vi "POM_PROM_host(1).vi"() -> ()   [LabVIEW 2013]
uses:
  <instrlib>/niDMM/nidmm.llb/niDMM Resolution in Digits.ctl
  <instrlib>/niDMM/nidmm.llb/niDMM Function.ctl
  <instrlib>/niDCPower/nidcpower.llb/niDCPower Measurement Type.ctl
  <vilib>/Analysis/baseanly.llb/Mean (DBL).vi
  <instrlib>/niDMM/nidmm.llb/niDMM Configure Measurement Digits.vi
  <vilib>/Analysis/NI_AALBase.lvlib
panel:
  in  "Принудительная стабилизация":bool
  out "I_pd, uA":dbl=291.5740420576185
  out "IPD(ext), mA":dbl=5.462609109167353
  out "IPD, mA":dbl(graph)=5.462609109167353
  out "Использовать Офир?":bool
  out "Monitor Current, uA":dbl(graph)=291.5700024459511
  in  "В ручную":bool
  in  "Напряжение Пельтье":dbl=0.8
  in  "Нагрев":bool
  in  "№#":i32=1802001
  out "Стабилизировано":bool=TRUE
  in  "+ V TEC для новой точки":dbl=0.11 format="%#_13g"
  in  "Вычет для \"антиразгона\"":dbl format="%#_13g"
  in  "Оставить в раб.\nрежиме":bool
  out "Boolean":bool
  in  "Num_hits_req":u64=5
  out "Num_hits":u64=371
  in  "Count_hits?":bool
  in  "tstab между точками, мс":u32=1
  in  "Предел тока PDext, мА":dbl=20.0
  in  "Dose":i32=7
  in  "Отладка(F)/\n/Рабочий(T)":bool=TRUE
  out "TEC_current, mA":dbl=186.4027731461029
  out "V2(Ild)_Log_address":refnum<file>
  out "Ipd(Ild)_External_Log_address":refnum<file>
  in  "Param_Log":path=path "D:/#rkm/Фонон-4/ТермоЛазер/Фонон-4_ПОМ_ПрОМ/Прога/Updated/ThermoLaser/Logs/Проверка/Проверка"
  out "Param_Log_address":refnum<file>
  out "Op(Ild)_Log_address":refnum<file>
  out "Ipd(Ild)_Monitor_Log_address":refnum<file>
  in  "trelax":u32=35000
  out "Volt_onRes":dbl=2.2062080678161866
  out "NoStab":bool
  out "Operating Current, mA":dbl=47.943356447720134
  in  "Desirable Operating current, mA":dbl=48.0 format="%#_6f"
  out "Error message":string
  in  "Up_Volt_limit":dbl=5.0
  in  "Low_Volt_limit":dbl=1.0
  out "ThRes_stabil":bool=TRUE
  out "Подстроенное напряжение\nстабилизации":dbl=0.7127853808593756
  out "ThRes value":dbl=17929.437890625
  in  "Optimum ThRes":dbl=18000.0 format="%#_6f"
  in  "Предел тока LD, мА":dbl=70.0
  in  "Предел тока ТЕС, мА":dbl=300.0
  in  "Tab Control":enum32{"Page 1", "Page 2", "Page 3", "Page 4"}(tab)=enum."Page 4"
  out "RES(U_TEC) Graph":cluster{dbl[], dbl[]}(graph)={[-0.0, 0.025, 0.05, 0.07500000000000001, 0.1, 0.125, 0.15, 0.175, 0.19999999999999998, 0.22499999999999998, 0.24999999999999997, 0.27499999999999997, 0.3, 0.325, 0.35000000000000003, 0.37500000000000006, 0.4000000000000001, 0.4250000000000001, 0.4500000000000001, 0.47500000000000014, 0.5000000000000001, 0.5250000000000001, 0.5500000000000002, 0.5750000000000002, 0.6000000000000002, 0.6250000000000002, 0.6500000000000002, 0.6750000000000003, 0.7000000000000003, 0.7250000000000003, 0.7500000000000003, 0.7750000000000004], [15319.04365234375, 15328.19267578125, 15358.49169921875, 15409.562109375, 15479.3826171875, 15563.1861328125, 15668.50888671875, 15780.12734375, 15906.40224609375, 16043.244921875, 16186.97255859375, 16341.84609375, 16507.0697265625, 16676.522265625, 16856.963671875, 17044.884375, 17239.0294921875, 17436.3736328125, 17641.744140625, 17850.8728515625, 18071.7896484375, 18291.20625, 18518.965625, 18750.4271484375, 18987.4517578125, 19230.0744140625, 19480.026171875, 19731.8517578125, 19984.940234375, 20249.54140625, 20514.206640625, 20780.055078125]}
  out "RES(I_TEC) Graph":cluster{dbl[], dbl[]}(graph)={[0.03457500435386299, 4.049114950716204, 7.9212407853678135, 11.611043015146826, 15.078954849250364, 18.53827902856892, 21.88408259580828, 25.295266856430793, 28.546483256934756, 31.60504570629327, 34.77027313644012, 37.80993408960394, 40.856486299311584, 43.94949565069024, 47.03219408159836, 50.06845592920464, 52.92926046093485, 55.95350027659507, 58.865931959242474, 61.84202368829837, 64.7802788203752, 67.60156326899994, 70.44177990185035, 73.41963022613506, 76.46974363403558, 79.22741287887104, 82.2001312992484, 85.07135997639818, 88.0785044464861, 90.98931976346292, 93.95691599392462, 96.75420696595256], [15319.04365234375, 15328.19267578125, 15358.49169921875, 15409.562109375, 15479.3826171875, 15563.1861328125, 15668.50888671875, 15780.12734375, 15906.40224609375, 16043.244921875, 16186.97255859375, 16341.84609375, 16507.0697265625, 16676.522265625, 16856.963671875, 17044.884375, 17239.0294921875, 17436.3736328125, 17641.744140625, 17850.8728515625, 18071.7896484375, 18291.20625, 18518.965625, 18750.4271484375, 18987.4517578125, 19230.0744140625, 19480.026171875, 19731.8517578125, 19984.940234375, 20249.54140625, 20514.206640625, 20780.055078125]}
  out "I_PD_Ext(I_LD) Graph":cluster{dbl[], dbl[]}(graph)={[0.0, 5.125820672560687, 10.202363077068034, 15.09070291650038, 20.026524721844005, 24.848748653112324, 29.706585438813228, 34.55255888002156, 39.41379829521783, 44.31743313126964, 49.35841653002704], [0.6213749657825949, 0.6126206411732633, 0.5986137214569519, 0.5846068013204628, 0.5933611264550083, 0.5670981505590477, 0.5355825775341941, 0.586357666360488, 0.5355825775341941, 0.5478386339632713, 0.5390843079753067]}
  out "I_PD(I_LD) Graph":cluster{dbl[], dbl[]}(graph)={[0.0, 5.125820672560687, 10.202363077068034, 15.09070291650038, 20.026524721844005, 24.848748653112324, 29.706585438813228, 34.55255888002156, 39.41379829521783, 44.31743313126964, 49.35841653002704], [0.00446055423708458, 0.1890051237296575, 1.3185992656872259, 47.69851657329127, 96.3842059718445, 145.3466946259141, 195.95923949964345, 243.1108383461833, 288.08951028622687, 334.6654470078647, 377.8655605856329]}
  out "I_pd, uA 2":dbl
  out "V2(I_LD) Graph":cluster{dbl[], dbl[]}(graph)={[0.0, 5.125820672560687, 10.202363077068034, 15.09070291650038, 20.026524721844005, 24.848748653112324, 29.706585438813228, 34.55255888002156, 39.41379829521783, 44.31743313126964, 49.35841653002704], [0.0006418486043783589, 1.1699665507043246, 1.452329111789965, 1.6798119558569469, 1.9201177244634586, 2.150803801269446, 2.3862573437846697, 2.612869753183121, 2.8439823589319366, 3.0683008415602466, 3.3013683877429134]}
  out "Forward Voltage, V":dbl
  out "OP(I_LD) Graph":cluster{dbl[], dbl[]}(graph)={[0.0, 5.125820672560687, 10.202363077068034, 15.09070291650038, 20.026524721844005, 24.848748653112324, 29.706585438813228, 34.55255888002156, 39.41379829521783, 44.31743313126964, 49.35841653002704], [0.0, 0.0, 0.02, 0.74, 1.5, 2.27, 3.0300000000000002, 3.8, 4.58, 5.33, 6.119999999999999]}
  out "Ophir, mW":dbl
  out "Пороговый ток":dbl
  out "Boolean 2":bool
  out "Сопротивление терморез-ра":dbl(graph)=16035.80078125
  out "thRes_adj":dbl=16035.80078125 format="%0.2f"
  in  "Source-Ohm w8":u32=1000
  in  "Coeff_High":dbl=90000.0 format="%#_13g"
  in  "Coeff_low":dbl=20000.0 format="%#_13g"
  in  "Coeff_thr":dbl=1500.0
  out "+Voltage\nrequired":dbl=0.0008410915798611111
  out "Разница ThRes":dbl=75.6982421875
  out "Operating Current":dbl(graph)=0.04003745256828817
  out "Optical Power":dbl(graph)
  out "accommodated voltage (out)":dbl=5.841436967760056
  in  "4070_Rele_source":enum16{"S2_Ch0", "S1_Ch2"}(ring)
  in  "the upper limit for the voltage_LD":dbl=6.0
  in  "the lower limit for the voltage_LD":dbl=1.0
  in  "Start voltage_LD":dbl=2.0 format="%#.7f"
  in  "accuracy_LD":dbl=0.01 step=0.01
  in  "Res_LD":dbl=50.0
  out "#Итерации":i32=31
  in  "TEC_Source":enum16{"S1_Ch2", "S2_Ch0", "S3_Ch1"}(ring)
  in  "Start voltage":dbl=0.1 format="%#.7f"
  in  "the upper limit for the voltage":dbl=1.2
  in  "the lower limit for the voltage":dbl
  in  "Точность ThRes":dbl=75.0 step=0.01
  out "Ro, Ом":dbl=15321.56484375
  in  "OphirLMMeasurementLib.ICoLMMeasurement":refnum<k7>
  out "hDevice":i32=1001
  out "Ophir_address":refnum<k7>
  in  "Power Enable":bool
  in  "4071(2)":refnum<k15>="PXI1Slot4_2"
  out "4071(2)_adress":refnum<k15>="PXI1Slot4_2 (12)" caption="4071(1)_out"
  in  "4071(1)":refnum<k15>="PXI1Slot5_2"
  out "4071(1)_adress":refnum<k15>="PXI1Slot5_2 (12)" caption="4071(1)_out"
  out "4070_address":refnum<k15>="PXI1Slot4_2 (12)" caption="4070_out"
  in  "4070":refnum<k15>="PXI1Slot4_2"
  in  "Source_3":refnum<k15>
  out "Source_3_Vcc_out":refnum<k15> caption="S_3_out"
  out "Source_2_Vcc_out":refnum<k15>="PXI1Slot6 (1)" caption="S_2_out"
  in  "Source_2":refnum<k15>="PXI1Slot6"
  out "Source_1_Vcc_out":refnum<k15>="PXI1Slot2_2 (1)" caption="S_1_out"
  in  "Source_1":refnum<k15>="PXI1Slot2_2"
  out "Прервать":bool=TRUE
  in  "milliseconds to wait":u32=2000
  in  "Шаг напр\nдля TEC, В":dbl=0.025
  in  "Начальное\nнапряжение TEC, В":dbl
  in  "кол-во точек для TEC":i32=32
  in  "stop":bool
  in  "Case":T1(ring)=enum."Quit"
  out "Выполняется":bool
  in  "Раб. режим LD":bool
  in  "Хар-ка TEC":bool
  in  "Хар-ки от I_LD":bool
  out "Status:":string="IDLE"
  out "Подстроенный ток, mA":dbl=43.94711423439531
  in  "Шаг, мА":dbl=5.0
  in  "Начальный ток, мА":dbl
  in  "Кол-во точек":i32=10
  # "20"
  # "7"
  # "5"
  # "0,15"
  # "Охлаждение"
  # "ток Пельтье во время стабилизации"
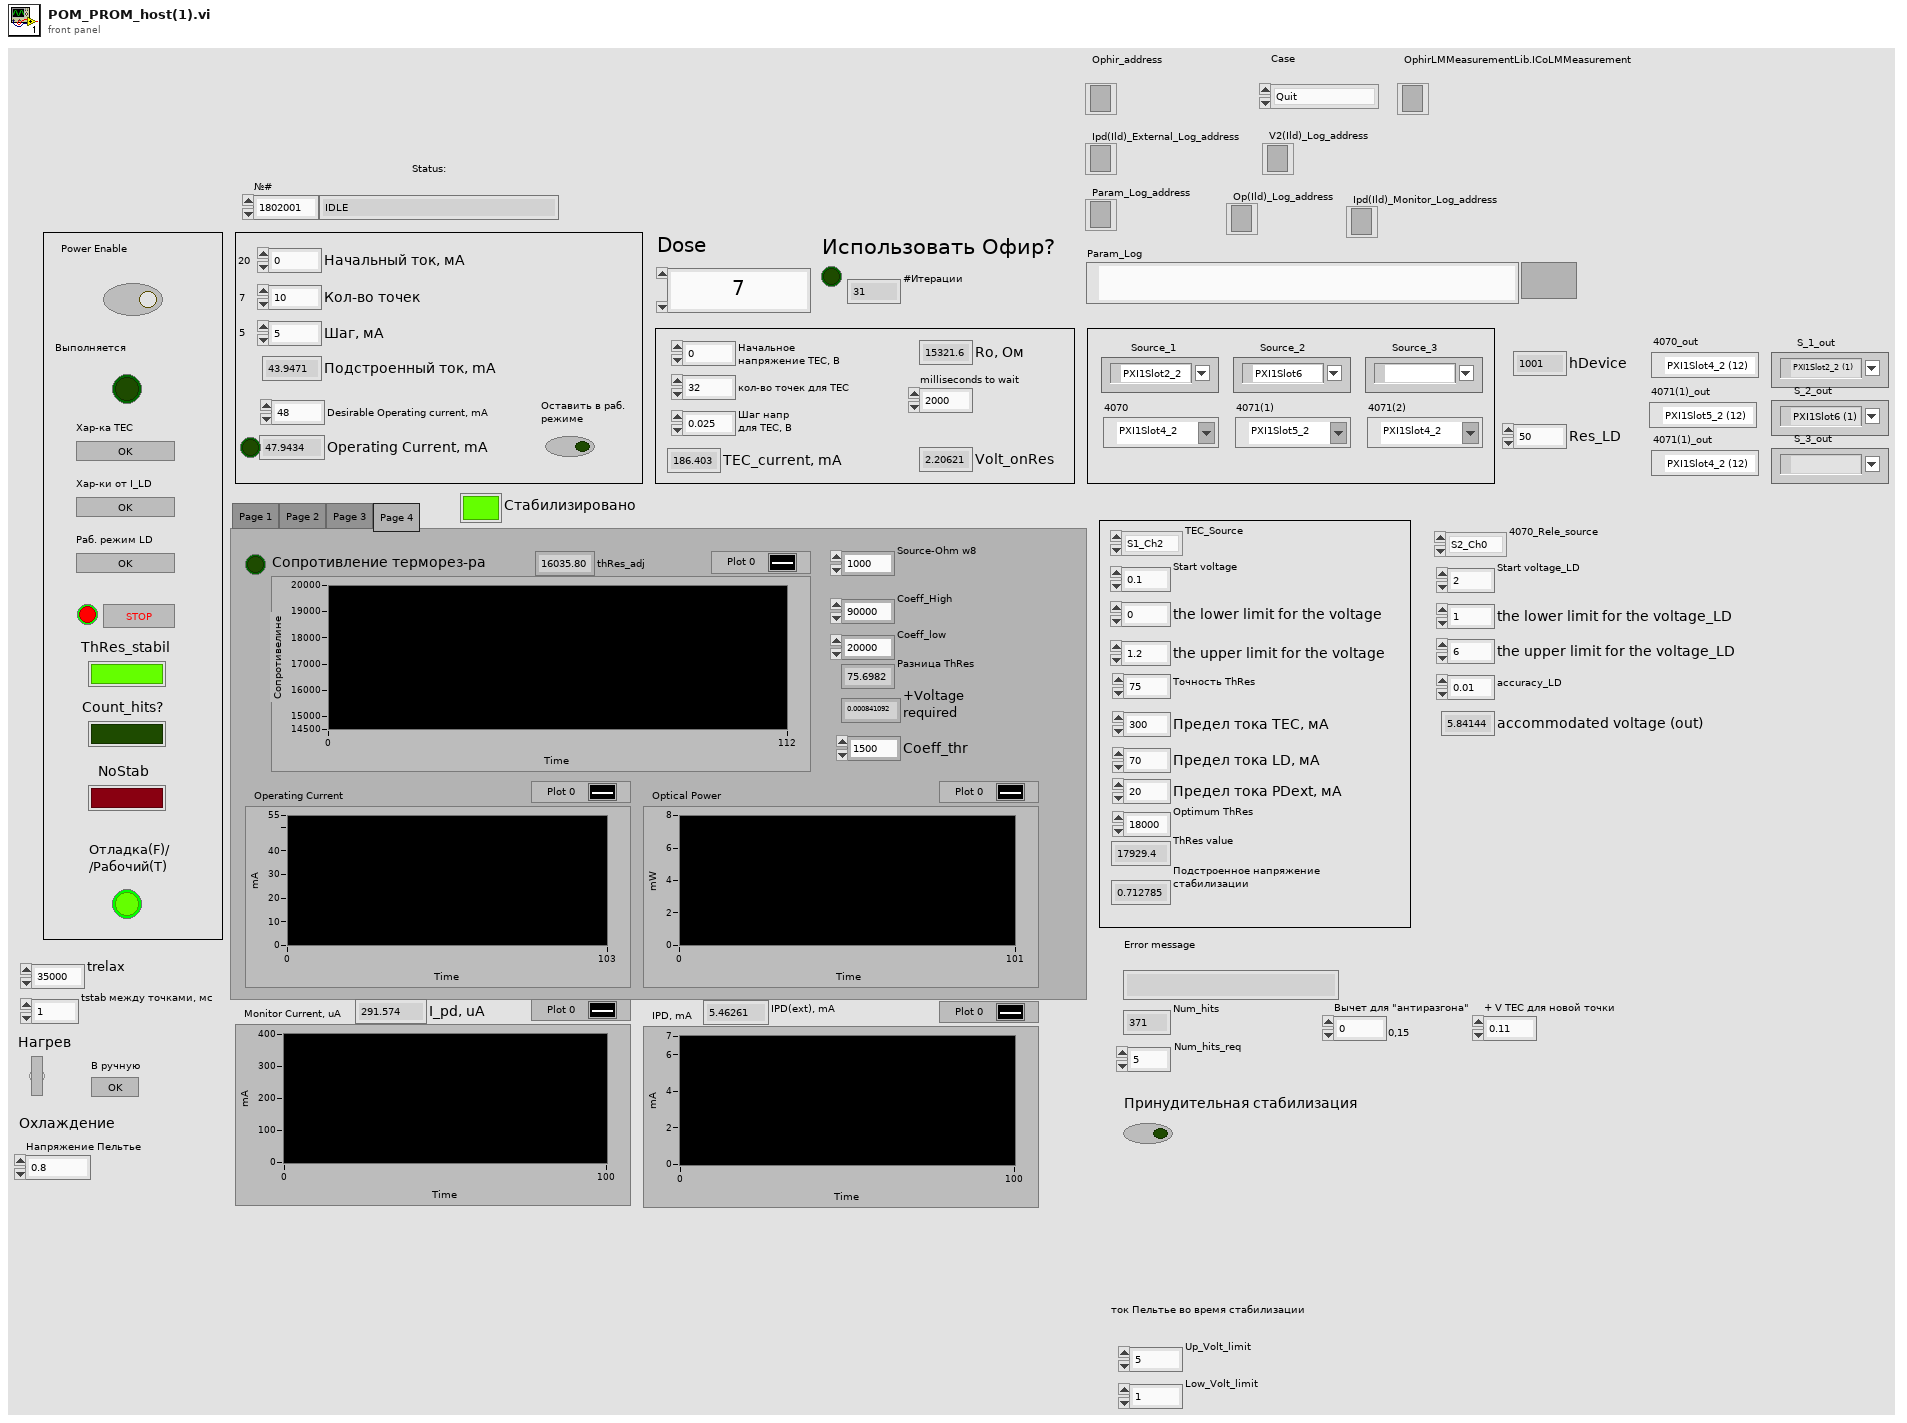
[diagram p1: front panel]
types:
  T1 = enum16{"Initialization", "TEC_Chars", "TRes_Check(Idle)", "Characteristics", "Bias", "Quit"}
  T2 = typedef "niDMM Function.ctl" = enum16{"DC Volts", "AC Volts", "DC Current", "AC Current", "2-wire Resistance", "4-wire Resistance", "Diode", "Frequency", "Period", "AC Volts DC Coupled", "Capacitance", "Inductance", "Temperature"}
  T3 = enum8{"Enabled", "Disabled", "Disabled and Grayed Out"}
  T4 = typedef "niDMM Resolution in Digits.ctl" = dbl
  T5 = enum16{"open", "replace", "create", "open or create", "replace or create", "replace or create with confirmation"}
  T6 = typedef "niDCPower Measurement Type.ctl" = i32
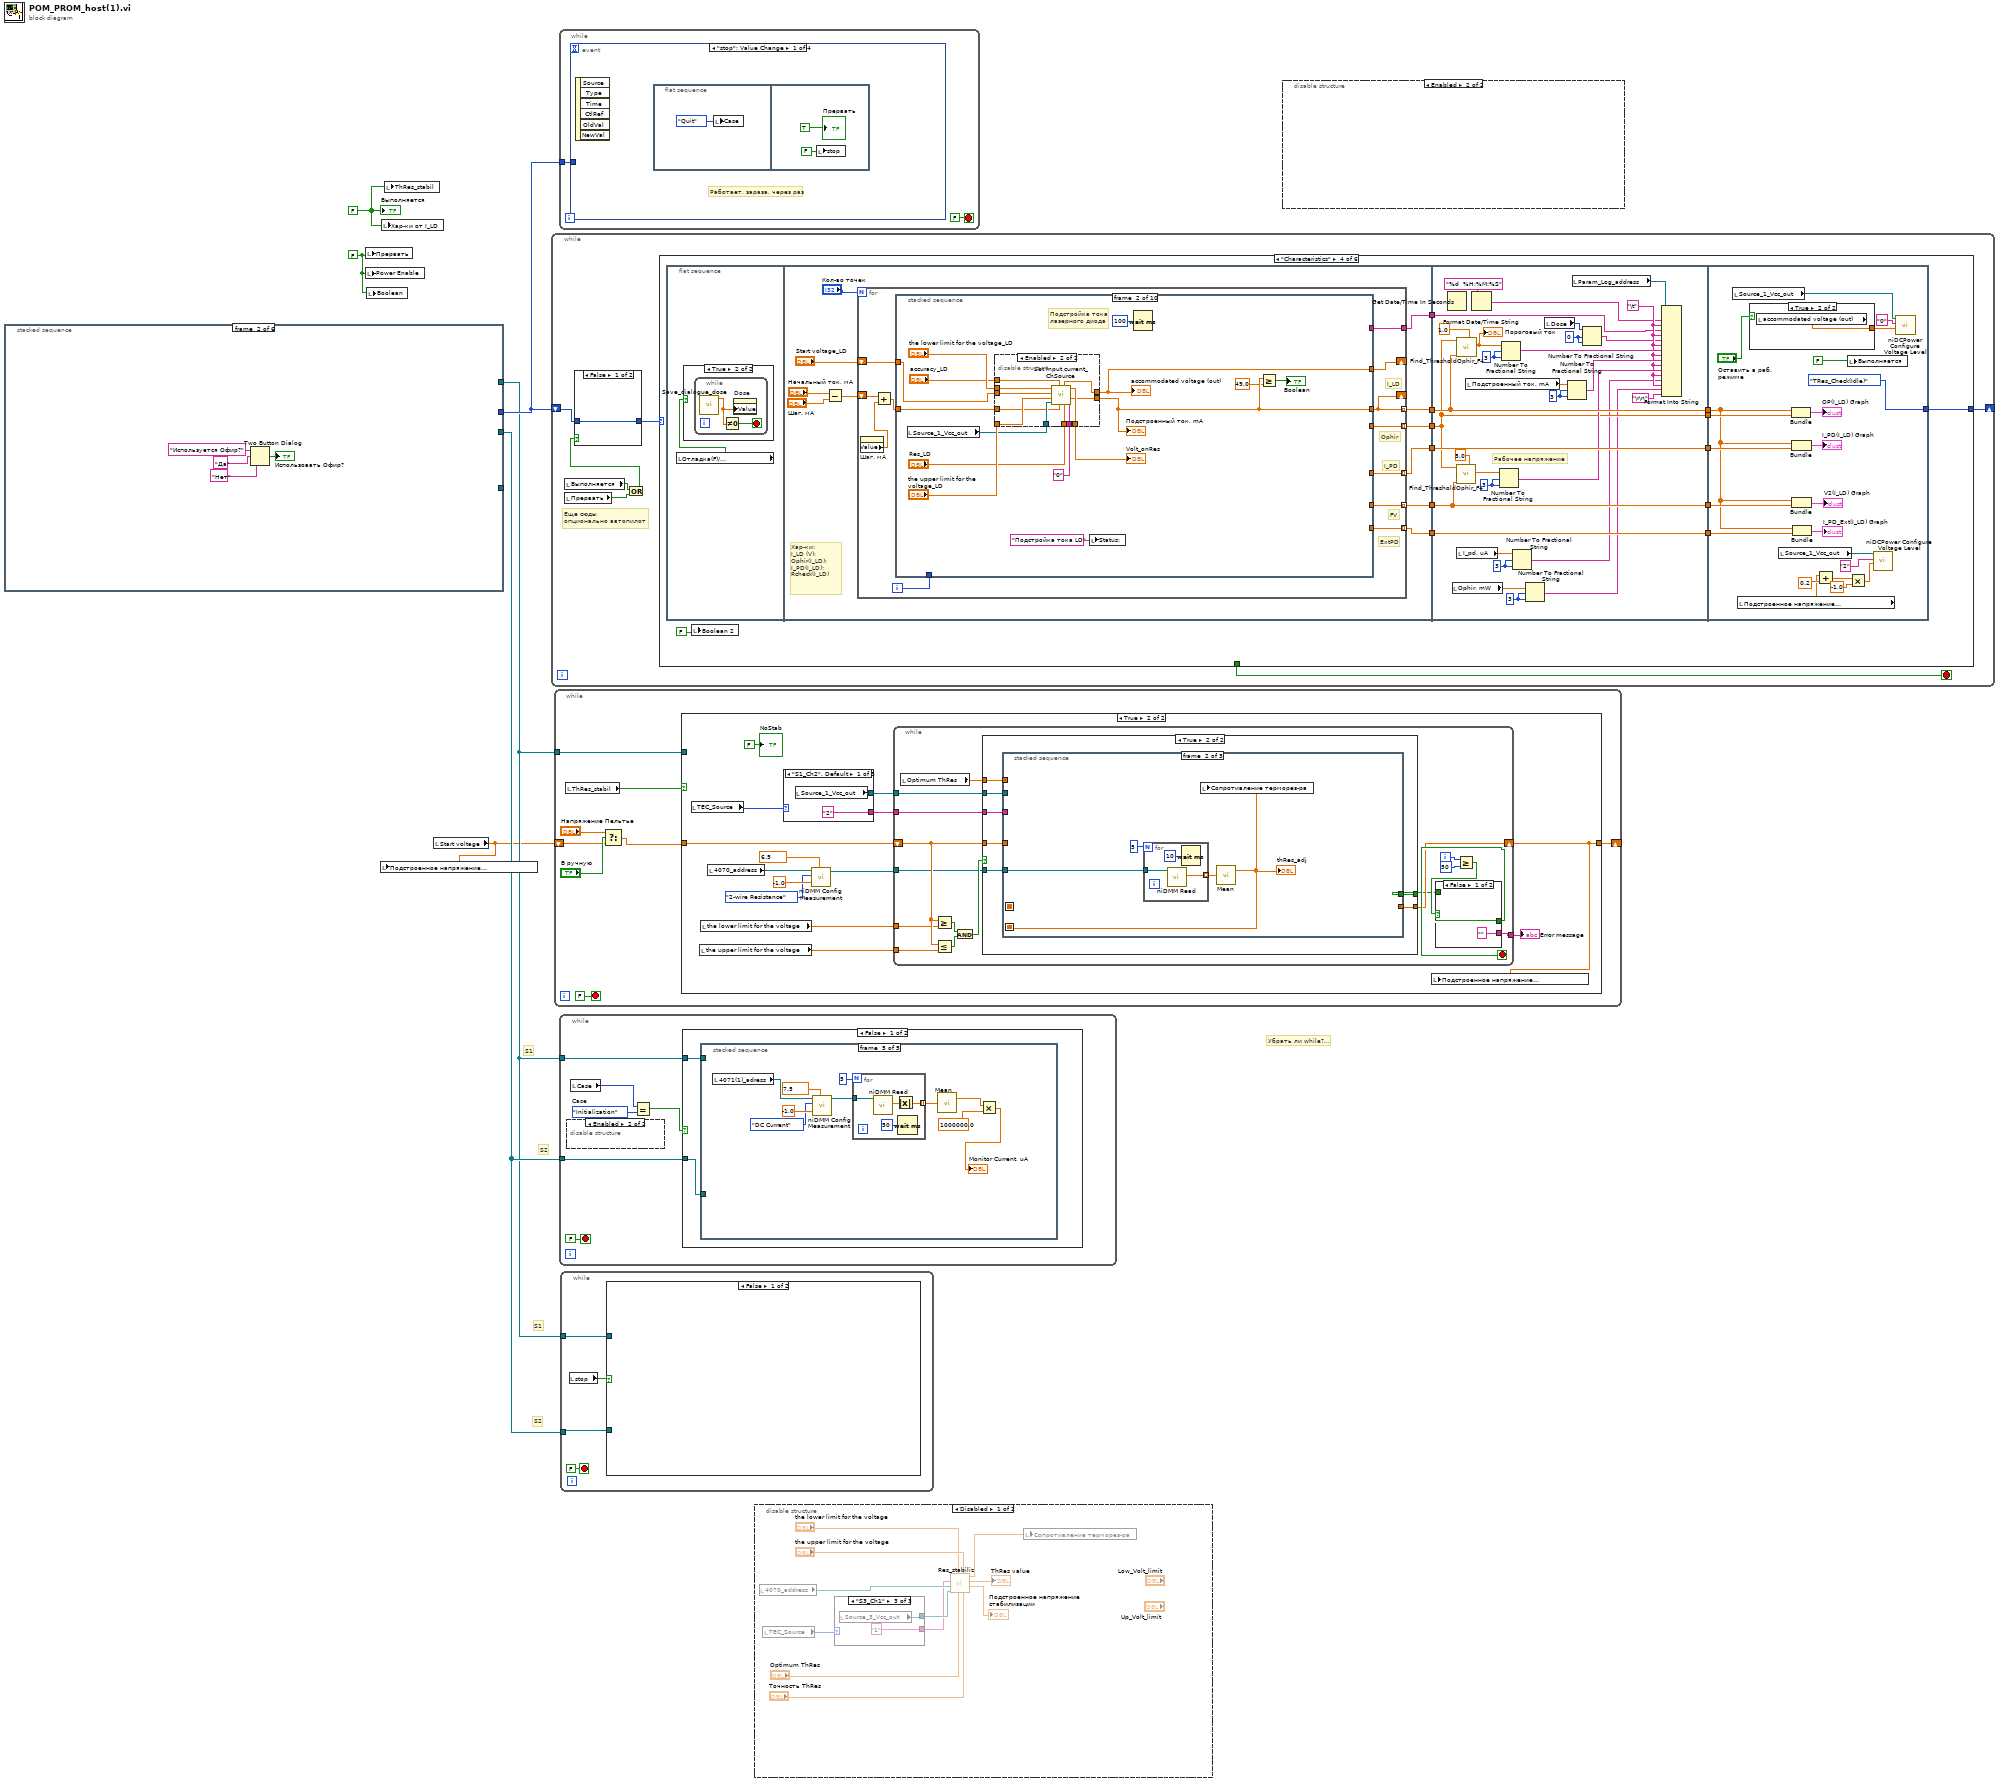
[diagram p0: block diagram]
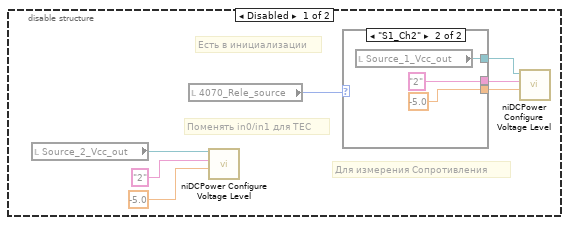
[diagram p2: hidden frame]
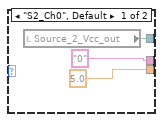
[diagram p3: hidden frame]
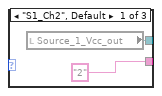
[diagram p4: hidden frame]
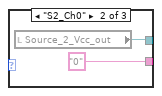
[diagram p5: hidden frame]
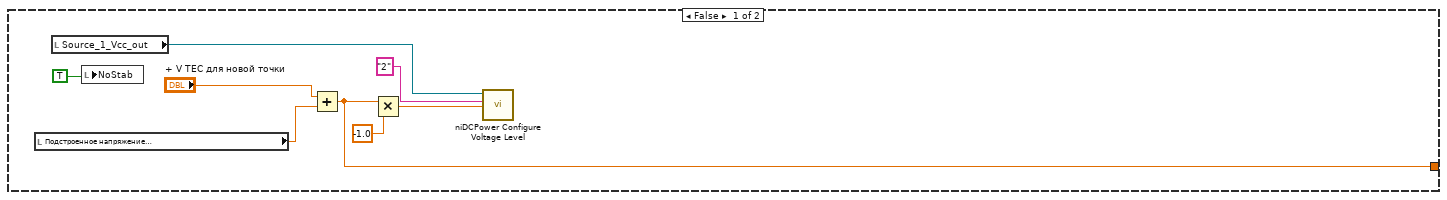
[diagram p7: hidden frame]
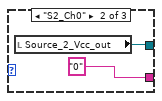
[diagram p8: hidden frame]
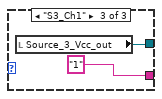
[diagram p9: hidden frame]
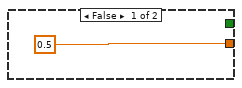
[diagram p10: hidden frame]
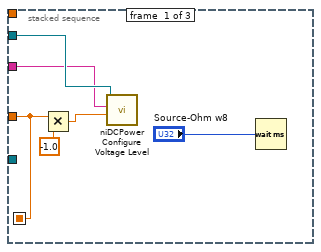
[diagram p11: hidden frame]
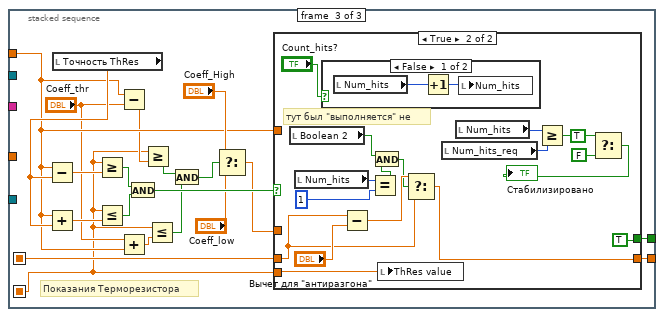
[diagram p12: hidden frame]
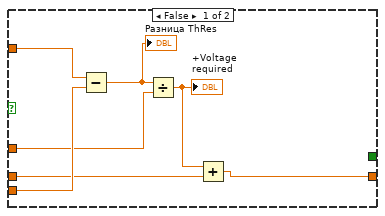
[diagram p13: hidden frame]
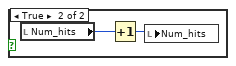
[diagram p14: hidden frame]
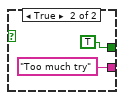
[diagram p15: hidden frame]
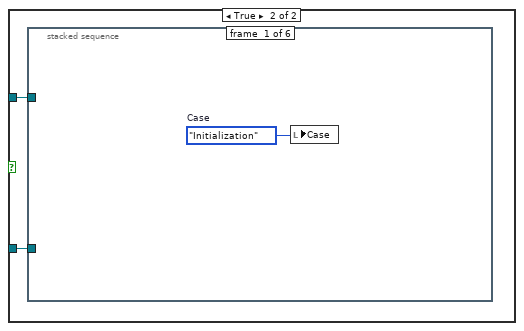
[diagram p16: hidden frame]
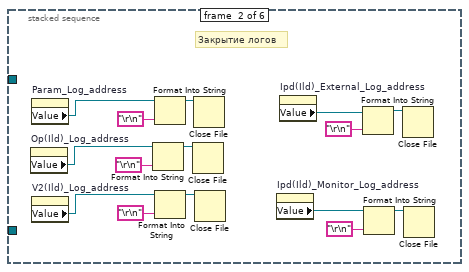
[diagram p17: hidden frame]
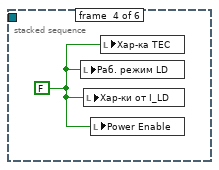
[diagram p19: hidden frame]
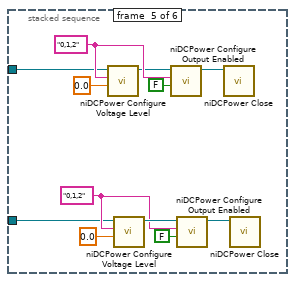
[diagram p20: hidden frame]
diagram:
  w4 = FALSE
  w2 = FALSE
  # "Убрать ли while?..."
  # "S1"
  # "S2"
  # "S2"
  # "S1"
  n1 = stacked-sequence {
    tunnel: [_ _ _ _ _ w88] -> w6
    tunnel: [_ _ w21 _ _ _] -> w5
    tunnel: [_ _ w20 _ _ _] -> w3
    tunnel: [_ _ w19 _ _ _] -> _
    frame #0 {
      n2 = while {
        stop <- w13 stop-if-true
        w8 = T3."Disabled and Grayed Out" ("Disabled")
        n3 = local write "Стабилизировано"(FALSE) -> ()
        n4 = property on="Хар-ка TEC" class="Bool (strict)"("DisabledEnum"=w8) -> ()  [unwired: 2 in, 2 out]
        n5 = property on="Раб. режим LD" class="Bool (strict)"("DisabledEnum"=w8) -> ()  [unwired: 2 in, 2 out]
        n6 = property on="Хар-ки от I_LD" class="Bool (strict)"("DisabledEnum"=w8) -> ()  [unwired: 2 in, 2 out]
        n7 = local write "Status:"("Ожидание Power Enable" ("Status:")) -> ()
        n8 = local read "stop"() -> (w11:bool)
        n9 = case shown="True" w11 {
          frame False {
          }
          frame True {
            n10 = local write "Прервать"(TRUE) -> ()
          }
        }
        n11 = Or(x=w11, y="Power Enable") -> (x .or. y?=w13:bool)
        n12 = Wait (ms)(milliseconds to wait=u32 100) -> ()  [unwired: 1 out]
      }
    }
    frame #1 {
      n13 = Two Button Dialog(message="Используется Офир?", 1:"Нет" ("F button name (\"Cancel\")"), 2:"Да" ("T button name (\"OK\")")) -> (T button?=→"Использовать Офир?":bool)
    }
    frame #2 {
      # "Источники"
      n14 = disable-structure shown="Enabled" {
        disable-tunnel: [w42 _] -> w19
        frame Disabled {
          n15 = call <instrlib>:"niDCPower Initialize.vi"("resource name"="Source_3") -> ("instrument handle out"=w46:refnum<k15>)  [unwired: 3 in, 7 out]
          n16 = call <instrlib>:"niDCPower Configure Voltage Level.vi"("voltage level"=0.0, "channel name"="0", "instrument handle"=w46) -> ("instrument handle out"=w45:refnum<k15>)  [unwired: 7 in, 1 out]
          n17 = call <instrlib>:"niDCPower Configure Voltage Level.vi"("voltage level"=0.0, "channel name"="1", "instrument handle"=w45) -> ("instrument handle out"=w51:refnum<k15>)  [unwired: 7 in, 1 out]
          n18 = call <instrlib>:"niDCPower Configure Voltage Level.vi"("voltage level"=0.0, "channel name"="2", "instrument handle"=w51) -> ("instrument handle out"=w42:refnum<k15>)  [unwired: 7 in, 1 out]
          "Source_3_Vcc_out" <- w42
        }
        frame Enabled {
        }
      }
      n19 = call <instrlib>:"niDCPower Initialize.vi"("resource name"="Source_1") -> ("instrument handle out"=w35:refnum<k15>)  [unwired: 3 in, 7 out]
      n20 = call <instrlib>:"niDCPower Initialize.vi"("resource name"="Source_2") -> ("instrument handle out"=w28:refnum<k15>)  [unwired: 3 in, 7 out]
      n21 = call <instrlib>:"niDCPower Configure Voltage Level.vi"("voltage level"=0.0, "channel name"="0", "instrument handle"=w35) -> ("instrument handle out"=w34:refnum<k15>)  [unwired: 7 in, 1 out]
      n22 = call <instrlib>:"niDCPower Configure Voltage Level.vi"("voltage level"=0.0, "channel name"="0", "instrument handle"=w28) -> ("instrument handle out"=w29:refnum<k15>)  [unwired: 7 in, 1 out]
      n23 = call <instrlib>:"niDCPower Configure Voltage Level.vi"("voltage level"=0.0, "channel name"="1", "instrument handle"=w34) -> ("instrument handle out"=w41:refnum<k15>)  [unwired: 7 in, 1 out]
      n24 = call <instrlib>:"niDCPower Configure Voltage Level.vi"("voltage level"=0.0, "channel name"="1", "instrument handle"=w29) -> ("instrument handle out"=w23:refnum<k15>)  [unwired: 7 in, 1 out]
      n25 = call <instrlib>:"niDCPower Configure Voltage Level.vi"("voltage level"=0.0, "channel name"="2", "instrument handle"=w41) -> ("instrument handle out"=w20:refnum<k15>)  [unwired: 7 in, 1 out]
      "Source_1_Vcc_out" <- w20
      n26 = call <instrlib>:"niDCPower Configure Voltage Level.vi"("voltage level"=0.0, "channel name"="2", "instrument handle"=w23) -> ("instrument handle out"=w21:refnum<k15>)  [unwired: 7 in, 1 out]
      "Source_2_Vcc_out" <- w21
    }
    frame #3 {
      w53 = T4 6.5 items=["3 1/2"=3.5, "4 1/2"=4.5, "5 1/2"=5.5, "6 1/2"=6.5, "7 1/2"=7.5] ("Resolution in Digits")
      w55 = TRUE ("Reset")
      (unwired) enum16{"S1_Ch2", "S2_Ch0", "S3_Ch1"}."S1_Ch2"  # TEC_Source
      w66 = T4 6.5 items=["3 1/2"=3.5, "4 1/2"=4.5, "5 1/2"=5.5, "6 1/2"=6.5, "7 1/2"=7.5] ("Resolution in Digits")
      w64 = TRUE ("Reset")
      # "4065"
      # "4070"
      # "Мультиметры"
      n27 = disable-structure shown="Disabled" {
        frame Disabled {
          w73 = T4 7.5 items=["3 1/2"=3.5, "4 1/2"=4.5, "5 1/2"=5.5, "6 1/2"=6.5, "7 1/2"=7.5] ("Resolution in Digits")
          w71 = TRUE ("Reset")
          # "4071"
          n28 = call <instrlib>:"niDMM Initialize.vi"("Reset"=w71, "ID Query"=w71, "Instrument Descriptor"="4071(2)") -> ("instrument handle out"=w69:refnum<k15>)  [unwired: 7 in, 1 out]
          n29 = call-poly <instrlib>:"niDMM Config Measurement.vi"("Range"=-1.0 ("Configuration:Measurement Options:Max Frequency"), "Resolution in Digits"=w73, "Function"=niDMM_Function."DC Current" ("multimeter mode"), "instrument handle"=w69) -> ("instrument handle out"=w67:refnum<k15>)  [unwired: 6 in, 1 out]
          "4071(2)_adress" <- w67
          n30 = call <instrlib>:"niDMM Read.vi"("instrument handle"=w67) -> ()  [unwired: 8 in, 3 out]
        }
        frame Enabled {
        }
      }
      n31 = call <instrlib>:"niDMM Initialize.vi"("Reset"=w55, "ID Query"=w55, "Instrument Descriptor"="4071(1)") -> ("instrument handle out"=w57:refnum<k15>)  [unwired: 7 in, 1 out]
      n32 = call <instrlib>:"niDMM Initialize.vi"("Reset"=w64, "ID Query"=w64, "Instrument Descriptor"="4070") -> ("instrument handle out"=w62:refnum<k15>)  [unwired: 7 in, 1 out]
      n33 = call-poly <instrlib>:"niDMM Config Measurement.vi"("Range"=-1.0 ("Configuration:Measurement Options:Max Frequency"), "Resolution in Digits"=w53, "Function"=niDMM_Function."DC Current" ("multimeter mode"), "instrument handle"=w57) -> ("instrument handle out"=w59:refnum<k15>)  [unwired: 6 in, 1 out]
      "4071(1)_adress" <- w59
      n34 = call-poly <instrlib>:"niDMM Config Measurement.vi"("Range"=-1.0 ("Configuration:Measurement Options:Max Frequency"), "Resolution in Digits"=w66, "Function"=niDMM_Function."DC Current" ("multimeter mode"), "instrument handle"=w62) -> ("instrument handle out"=w60:refnum<k15>)  [unwired: 6 in, 1 out]
      "4070_address" <- w60
      n35 = call <instrlib>:"niDMM Read.vi"("instrument handle"=w59) -> ()  [unwired: 8 in, 3 out]
      n36 = call <instrlib>:"niDMM Read.vi"("instrument handle"=w60) -> ()  [unwired: 8 in, 3 out]
    }
    frame #4 {
      n37 = local read "Использовать Офир?"() -> (w74:bool)
      n38 = case shown="True" w74 {
        frame False {
        }
        frame True {
          n39 = Automation Open(Automation Refnum="OphirLMMeasurementLib.ICoLMMeasurement") -> (Automation Refnum=w83:refnum<k7>)  [unwired: 3 in, 1 out]
          n40 = invoke class="ICoLMMeasurement" method="ScanUSB"(reference=w83) -> (reference out=w85:refnum<k7>, "serialNumbers"=w82:variant)  [unwired: 3 in, 2 out]
          "Ophir_address" <- w85
          n41 = Variant To Data(type=string[] [], Variant=w82) -> (data=w81:string[])  [unwired: 1 in, 1 out]
          n42 = Index Array(array=w81, index=0) -> (element=w78:string)
          n43 = invoke class="ICoLMMeasurement" method="OpenUSBDevice"(reference=w85, "serialNumber"=w78) -> (reference out=w77:refnum<k7>, "hDevice"=w76:i32)  [unwired: 3 in, 3 out]
          "hDevice" <- w76
          n44 = invoke class="ICoLMMeasurement" method="StartStream"(reference=w77, "hDevice"=w76, "channel"=0) -> ()  [unwired: 2 in, 5 out]
        }
      }
    }
    frame #5 {
      (unwired) enum16{"S2_Ch0", "S1_Ch2"}."S2_Ch0"  # 4070_Rele_source
      w88 = T1."Initialization"  # Case
      n45 = property on="Сопротивление терморез-ра" class="WFChart (strict)"("History Data"=dbl[] []) -> ()  [unwired: 2 in, 2 out]
      n46 = local write "Start voltage"("Start voltage") -> ()
    }
  }
  n47 = local write "Прервать"(w2) -> ()
  n48 = local write "Power Enable"(w2) -> ()
  n49 = local write "Boolean"(w2) -> ()
  n50 = local write "Хар-ки от I_LD"(w4) -> ()
  n51 = local write "ThRes_stabil"(w4) -> ()
  n52 = local read "Start voltage"() -> (w1:dbl)
  n53 = local write "Подстроенное напряжение\nстабилизации"(w1) -> ()
  n54 = while {
    shift-right: [w89] -> _
    shift-left: w6 -> [w95]
    stop <- w93 stop-if-true
    # "Еще сюды\nопционально автопилот"
    n55 = local read "Выполняется"() -> (w92:bool)
    n56 = local read "Прервать"() -> (w91:bool)
    n57 = Or(x=w92, y=w91) -> (x .or. y?=w90:bool)
    n58 = case shown="False" w90 {
      tunnel: w95 -> [w96 _]
      tunnel: [w96 "Case"] -> w94
      frame False {
      }
      frame True {
      }
    }
    n59 = case shown="\"Characteristics\"" w94 {
      tunnel: [_ _ _ _ _ TRUE] -> w93
      tunnel: [w98 w225 w394 w434 w726 T1."Quit" ("Case")] -> w89
      frame "Initialization", Default {
        n60 = stacked-sequence {
          tunnel: [_ _ _ _ T1."TRes_Check(Idle)" ("Case")] -> w98
          frame #0 {
            w101 = T3."Enabled" ("Disabled")
            n61 = property on="Хар-ка TEC" class="Bool (strict)"("DisabledEnum"=w101) -> ()  [unwired: 2 in, 2 out]
            n62 = property on="Раб. режим LD" class="Bool (strict)"("DisabledEnum"=w101) -> ()  [unwired: 2 in, 2 out]
            n63 = property on="Хар-ки от I_LD" class="Bool (strict)"("DisabledEnum"=w101) -> ()  [unwired: 2 in, 2 out]
          }
          frame #1 {
            # "Питание внешнего фотодиода"
            # "Поменять in0/in1 для ТЕС"
            # "Режим омметра"
            n64 = local read "4070_Rele_source"() -> (w109:enum16{"S2_Ch0", "S1_Ch2"})
            n65 = local read "Source_2_Vcc_out"() -> (w107:refnum<k15>)
            n66 = local read "Source_2_Vcc_out"() -> (w104:refnum<k15>)
            n67 = case shown="\"S2_Ch0\", Default" w109 {
              tunnel: [5.0 -5.0] -> w110
              tunnel: ["0" "2"] -> w111
              tunnel: [w113 w116] -> w112
              frame "S2_Ch0", Default {
                n68 = local read "Source_2_Vcc_out"() -> (w113:refnum<k15>)
              }
              frame "S1_Ch2" {
                n69 = local read "Source_1_Vcc_out"() -> (w116:refnum<k15>)
              }
            }
            n70 = call <instrlib>:"niDCPower Configure Voltage Level.vi"("voltage level"=-5.0, "channel name"="2", "instrument handle"=w107) -> ()  [unwired: 7 in, 2 out]
            n71 = call <instrlib>:"niDCPower Configure Voltage Level.vi"("voltage level"=5.0, "channel name"="1", "instrument handle"=w104) -> ()  [unwired: 7 in, 2 out]
            n72 = call <instrlib>:"niDCPower Configure Voltage Level.vi"("voltage level"=w110, "channel name"=w111, "instrument handle"=w112) -> ()  [unwired: 7 in, 2 out]
            n73 = Wait (ms)(milliseconds to wait=u32 500) -> ()  [unwired: 1 out]
          }
          frame #2 {
            w121 = FALSE
            n74 = local write "NoStab"(w121) -> ()
            n75 = local write "Count_hits?"(w121) -> ()
            n76 = local write "Num_hits"(u64 0 ("Num_hits")) -> ()
            "ThRes_stabil" <- TRUE
            "Boolean 2" <- TRUE
          }
          frame #3 {
            w134 = "\t"
            w150 = "\t"
            w206 = "\t"
            w210 = "\t"
            w167 = "\t"
            n77 = Number To Fractional String(number="№#", width (-)=i16 7, precision (6)=i16 0) -> (F-format string=w142:string)  [unwired: 1 in]
            n78 = Build Path(base path="Param_Log", name or relative path=w142) -> (appended path=w177:path)
            n79 = call <vilib>:"Check if File or Folder Exists.vi"("path"=w177) -> ("file or folder exists?"=w175:bool, "dup path"=w176:path)  [unwired: 8 in, 1 out]
            n80 = Concatenate Strings(w142, "_" ("element"), "Param_log" ("string"), ".txt" ("element")) -> (w171:string)
            n81 = Concatenate Strings(w142, "_" ("element"), "Op(Ild)_log" ("string"), ".txt" ("element")) -> (w186:string)
            n82 = Concatenate Strings(w142, "_" ("element"), "Ipd(Ild)_Monitor_log" ("string"), ".txt" ("element")) -> (w197:string)
            n83 = Concatenate Strings(w142, "_" ("element"), "Ipd(Ild)_External_log" ("string"), ".txt" ("element")) -> (w156:string)
            n84 = Concatenate Strings(w142, "_" ("element"), "V2(Ild)_log" ("string"), ".txt" ("element")) -> (w138:string)
            n85 = case shown="False" w175 {
              tunnel: w176 -> [w222 w223]
              tunnel: [w221 w223] -> w127
              frame False {
                n86 = Create Folder(path (use dialog)=w222) -> (created path=w221:path)  [unwired: 2 in, 2 out]
              }
              frame True {
              }
            }
            n87 = Build Path(base path=w127, name or relative path=w171) -> (appended path=w172:path)
            n88 = Build Path(base path=w127, name or relative path=w138) -> (appended path=w140:path)
            n89 = Build Path(base path=w127, name or relative path=w186) -> (appended path=w188:path)
            n90 = Build Path(base path=w127, name or relative path=w197) -> (appended path=w192:path)
            n91 = Build Path(base path=w127, name or relative path=w156) -> (appended path=w158:path)
            n92 = Open/Create/Replace File(file path (use dialog)=w172, operation (0:open)=T5."open or create", access (0:read/write)=enum16{"read/write", "read-only", "write-only"}."read/write") -> (refnum out=w165:refnum<file>)  [unwired: 3 in, 2 out]
            "Param_Log_address" <- w165
            n93 = Open/Create/Replace File(file path (use dialog)=w188, operation (0:open)=T5."open or create", access (0:read/write)=enum16{"read/write", "read-only", "write-only"}."read/write") -> (refnum out=w166:refnum<file>)  [unwired: 3 in, 2 out]
            "Op(Ild)_Log_address" <- w166
            n94 = Open/Create/Replace File(file path (use dialog)=w140, operation (0:open)=T5."open or create", access (0:read/write)=enum16{"read/write", "read-only", "write-only"}."read/write") -> (refnum out=w128:refnum<file>)  [unwired: 3 in, 2 out]
            "V2(Ild)_Log_address" <- w128
            n95 = Open/Create/Replace File(file path (use dialog)=w192, operation (0:open)=T5."open or create", access (0:read/write)=enum16{"read/write", "read-only", "write-only"}."read/write") -> (refnum out=w203:refnum<file>)  [unwired: 3 in, 2 out]
            "Ipd(Ild)_Monitor_Log_address" <- w203
            n96 = Open/Create/Replace File(file path (use dialog)=w158, operation (0:open)=T5."open or create", access (0:read/write)=enum16{"read/write", "read-only", "write-only"}."read/write") -> (refnum out=w146:refnum<file>)  [unwired: 3 in, 2 out]
            "Ipd(Ild)_External_Log_address" <- w146
            n97 = Format Into String(initial string=w165, "Time" ("input 1"), w167, "Mode" ("input 6"), w167, "Dose" ("input 1"), w167, "Thr_Cur, mA" ("input 6"), w167, "Op_Cur, mA " ("input 6"), w167, "Op_Vol, V" ("input 6"), w167, "Ipd, uA" ("input 6"), w167, "OutPow, mW" ("input 6"), w167, "Dark_Cur, uA" ("input 6"), "\r\n") -> (resulting string=w178:refnum<file>)  [unwired: 2 in, 1 out]
            n98 = Format Into String(initial string=w203, "Time" ("input 1"), w206, "Mode" ("input 6"), w206, "Dose" ("input 1"), w206, "Ild, mA" ("input 6"), w206, "Ipd, uA" ("input 6"), w206, "\r\n") -> (resulting string=w200:refnum<file>)  [unwired: 2 in, 1 out]
            n99 = Format Into String(initial string=w128, "Time" ("input 1"), w134, "Mode" ("input 6"), w134, "Dose" ("input 1"), w134, "Ild, mA" ("input 6"), w134, "V2, V" ("input 6"), w134, "\r\n") -> (resulting string=w129:refnum<file>)  [unwired: 2 in, 1 out]
            n100 = Set File Position(refnum=w200, from (0:start)=enum16{"start", "end", "current"}."end") -> ()  [unwired: 2 in, 2 out]
            n101 = Set File Position(refnum=w129, from (0:start)=enum16{"start", "end", "current"}."end") -> ()  [unwired: 2 in, 2 out]
            n102 = Set File Position(refnum=w178, from (0:start)=enum16{"start", "end", "current"}."end") -> ()  [unwired: 2 in, 2 out]
            n103 = Format Into String(initial string=w166, "Time" ("input 1"), w210, "Mode" ("input 6"), w210, "Dose" ("input 1"), w210, "Ild, mA" ("input 6"), w210, "Op, mW" ("input 6"), "\r\n") -> (resulting string=w199:refnum<file>)  [unwired: 2 in, 1 out]
            n104 = Format Into String(initial string=w146, "Time" ("input 1"), w150, "Mode" ("input 6"), w150, "Dose" ("input 1"), w150, "Ild, mA" ("input 6"), w150, "IPD, mA" ("input 6"), w150, "\r\n") -> (resulting string=w155:refnum<file>)  [unwired: 2 in, 1 out]
            n105 = Set File Position(refnum=w199, from (0:start)=enum16{"start", "end", "current"}."end") -> ()  [unwired: 2 in, 2 out]
            n106 = Set File Position(refnum=w155, from (0:start)=enum16{"start", "end", "current"}."end") -> ()  [unwired: 2 in, 2 out]
          }
          frame #4 {
          }
        }
        n107 = Wait (ms)(milliseconds to wait=u32 100) -> ()  [unwired: 1 out]
        "Status:" <- "Инициализация" ("Status:")
      }
      frame "TEC_Chars" {
        n108 = while {
          tunnel: [w227] -> w225
          stop <- w226 stop-if-true
          n109 = stacked-sequence {
            tunnel: [_ _ w273 _] -> w227
            tunnel: [_ _ w271 _] -> w226
            frame #0 {
              n110 = local write "Boolean 2"(FALSE) -> ()
              n111 = stacked-sequence {
                frame #0 {
                  # "Переключение в режим Омметра"
                  n112 = local read "4070_Rele_source"() -> (w233:enum16{"S2_Ch0", "S1_Ch2"})
                  n113 = case shown="\"S2_Ch0\", Default" w233 {
                    tunnel: [5.0 -5.0] -> w232
                    tunnel: ["0" "2"] -> w231
                    tunnel: [w234 w237] -> w230
                    frame "S2_Ch0", Default {
                      n114 = local read "Source_2_Vcc_out"() -> (w234:refnum<k15>)
                    }
                    frame "S1_Ch2" {
                      n115 = local read "Source_1_Vcc_out"() -> (w237:refnum<k15>)
                    }
                  }
                  n116 = call <instrlib>:"niDCPower Configure Voltage Level.vi"("voltage level"=w232, "channel name"=w231, "instrument handle"=w230) -> ()  [unwired: 7 in, 2 out]
                }
                frame #1 {
                  w240 = FALSE
                  # "Отключение стабилизации"
                  n117 = while {
                    tunnel: w240 -> [_]
                    stop <- w241 stop-if-true
                    n118 = local read "NoStab"() -> (w241:bool)
                  }
                  n119 = local write "ThRes_stabil"(w240) -> ()
                }
                frame #2 {
                  # "Перестановка in0 и in1 (+ и - у Пельтье)"
                  n120 = local read "Source_2_Vcc_out"() -> (w243:refnum<k15>)
                  n121 = call <instrlib>:"niDCPower Configure Voltage Level.vi"("voltage level"=-5.0, "channel name"="2", "instrument handle"=w243) -> ()  [unwired: 7 in, 2 out]
                }
                frame #3 {
                  # "Отключение пельтье"
                  n122 = local read "Source_1_Vcc_out"() -> (w245:refnum<k15>)
                  n123 = call <instrlib>:"niDCPower Configure Voltage Level.vi"("voltage level"=0.0, "channel name"="2", "instrument handle"=w245) -> ()  [unwired: 7 in, 2 out]
                }
                frame #4 {
                  n124 = Wait (ms)(milliseconds to wait="trelax") -> ()  [unwired: 1 out]
                }
              }
              n125 = local write "Status:"("Выравнивание температуры" ("Status:")) -> ()
            }
            frame #1 {
              w256 = T4 6.5 items=["3 1/2"=3.5, "4 1/2"=4.5, "5 1/2"=5.5, "6 1/2"=6.5, "7 1/2"=7.5] ("Resolution in Digits")
              n126 = local write "Выполняется"(TRUE) -> ()
              n127 = local read "4070_address"() -> (w255:refnum<k15>)
              n128 = call-poly <instrlib>:"niDMM Config Measurement.vi"("Range"=-1.0 ("Configuration:Measurement Options:Max Frequency"), "Resolution in Digits"=w256, "Function"=niDMM_Function."2-wire Resistance" ("multimeter mode"), "instrument handle"=w255) -> ("instrument handle out"=w252:refnum<k15>)  [unwired: 6 in, 1 out]
              n129 = for {
                N: 2 -> [_]
                tunnel: w252 -> [w262]
                tunnel: [w261] -> w251
                n130 = call <instrlib>:"niDMM Read.vi"("instrument handle"=w262) -> ("instrument handle out"=w261:refnum<k15>)  [unwired: 8 in, 2 out]
              }
              n131 = for {
                N: 5 -> [_]
                tunnel: w251 -> [w264]
                tunnel: [w263] -> w254 mode=indexing
                n132 = call <instrlib>:"niDMM Read.vi"("instrument handle"=w264) -> ("Measurement"=w263:dbl)  [unwired: 8 in, 2 out]
                n133 = Wait (ms)(milliseconds to wait=u32 100) -> ()  [unwired: 1 out]
              }
              n134 = call-poly <vilib>:"Mean.vi"("X"=w254) -> ("mean"=→"Ro, Ом":dbl)  [unwired: 1 out]
              n135 = local write "Status:"("Измерение сопротивления в отсутствии тока " ("Status:")) -> ()
            }
            frame #2 {
              # "Подстройка тока\nдля пельтье"
              # "При достижении 0V поменять\nполярность, поменяв направление\nтока с помощью реле"
              n136 = Add(x="Начальное\nнапряжение TEC, В", y="Шаг напр\nдля TEC, В") -> (x+y=w266:dbl)
              n137 = for {
                N: "кол-во точек для TEC" -> [_]
                tunnel: [w296] -> w268 mode=indexing
                tunnel: [w295] -> w270 mode=indexing
                tunnel: "Шаг напр\nдля TEC, В" -> [w292]
                tunnel: [w291] -> w267 mode=indexing
                shift-right: [w294] -> _
                shift-left: w266 -> [w293]
                i -> [w290]
                # "R"
                # "I"
                # "V"
                n138 = stacked-sequence {
                  seq-local: [w298 _ _] -> [_ w327 _]
                  tunnel: [_ w328 _] -> w295
                  tunnel: [_ _ w356] -> w296
                  tunnel: [_ w327 _] -> w294
                  tunnel: w293 -> [w300 _ _]
                  tunnel: w292 -> [w299 _ _]
                  tunnel: [w297 _ _] -> w291
                  frame #0 {
                    n139 = disable-structure shown="Enabled" {
                      disable-tunnel: w300 -> [w305 w324]
                      disable-tunnel: w299 -> [w304 w325]
                      disable-tunnel: [w303 w323] -> w298
                      disable-tunnel: [w302 w322] -> w297
                      frame Disabled {
                        n140 = local read "кол-во точек для TEC"() -> (w310:i32)
                        n141 = local read "#Итерации"() -> (w307:i32)
                        n142 = Divide(x=w310, y=2) -> (x/y=w308:dbl)
                        n143 = Less?(x=w308, y=w307) -> (x < y?=w306:bool)
                        n144 = case shown="False" w306 {
                          tunnel: [0.0 -5.0] -> w311
                          tunnel: w305 -> [w314 w320]
                          tunnel: w304 -> [w313 w319]
                          tunnel: [w312 w318] -> w303
                          tunnel: [w312 w316] -> w302
                          frame False {
                            n145 = Add(x=w314, y=w313) -> (x+y=w312:dbl)
                          }
                          frame True {
                            n146 = Subtract(x=w320, y=w319) -> (x-y=w318:dbl)
                            n147 = Multiply(x=-1.0, y=w318) -> (x*y=w316:dbl)
                          }
                        }
                      }
                      frame Enabled {
                        n148 = Subtract(x=w324, y=w325) -> (x-y=w323:dbl)
                        n149 = Multiply(x=-1.0, y=w323) -> (x*y=w322:dbl)
                      }
                    }
                    n150 = Wait (ms)(milliseconds to wait=u32 100) -> ()  [unwired: 1 out]
                  }
                  frame #1 {
                    n151 = case shown="\"S1_Ch2\", Default" "TEC_Source" {
                      tunnel: [w351 w353 w355] -> w330
                      tunnel: ["2" "0" "1"] -> w329
                      frame "S1_Ch2", Default {
                        n152 = local read "Source_1_Vcc_out"() -> (w351:refnum<k15>)
                      }
                      frame "S2_Ch0" {
                        n153 = local read "Source_2_Vcc_out"() -> (w353:refnum<k15>)
                      }
                      frame "S3_Ch1" {
                        n154 = local read "Source_3_Vcc_out"() -> (w355:refnum<k15>)
                      }
                    }
                    n155 = flat-sequence {
                      tunnel: [w339] -> w334
                      tunnel: [w336] -> w333
                      tunnel: w330 -> [w338]
                      tunnel: w329 -> [w336]
                      tunnel: w327 -> [w337]
                      tunnel: w334 -> [w340]
                      tunnel: w333 -> [w341]
                      tunnel: [w341] -> w332
                      tunnel: [w340] -> w331
                      tunnel: w332 -> [w346]
                      tunnel: w331 -> [w347]
                      tunnel: [w349] -> w328
                      frame #0 {
                        n156 = call <instrlib>:"niDCPower Configure Voltage Level.vi"("voltage level"=w337, "channel name"=w336, "instrument handle"=w338) -> ("instrument handle out"=w339:refnum<k15>)  [unwired: 7 in, 1 out]
                      }
                      frame #1 {
                        n157 = Wait (ms)(milliseconds to wait=u32 100) -> ()  [unwired: 1 out]
                      }
                      frame #2 {
                        w348 = T6 0 items=["Current", "Voltage"] ("measurement type")
                        n158 = call <instrlib>:"niDCPower Measure.vi"("measurement type"=w348, "channel name"=w346, "instrument handle"=w347) -> ("measurement"=w345:dbl)  [unwired: 6 in, 2 out]
                        n159 = Multiply(x=w345, y=1000.0) -> (x*y=w343:dbl)
                        n160 = Absolute Value(x=w343) -> (abs(x)=w349:dbl)
                        "TEC_current, mA" <- w349
                      }
                    }
                  }
                  frame #2 {
                    w361 = T4 6.5 items=["3 1/2"=3.5, "4 1/2"=4.5, "5 1/2"=5.5, "6 1/2"=6.5, "7 1/2"=7.5] ("Resolution in Digits")
                    # "Снятие показаний\nТерморезистора"
                    n161 = local read "4070_address"() -> (w360:refnum<k15>)
                    n162 = call-poly <instrlib>:"niDMM Config Measurement.vi"("Range"=-1.0 ("Configuration:Measurement Options:Max Frequency"), "Resolution in Digits"=w361, "Function"=niDMM_Function."2-wire Resistance" ("multimeter mode"), "instrument handle"=w360) -> ("instrument handle out"=w359:refnum<k15>)  [unwired: 6 in, 1 out]
                    n163 = for {
                      N: 10 -> [_]
                      tunnel: w359 -> [w365]
                      tunnel: [w364] -> w358 mode=indexing
                      n164 = call <instrlib>:"niDMM Read.vi"("instrument handle"=w365) -> ("Measurement"=w364:dbl)  [unwired: 8 in, 2 out]
                      n165 = Wait (ms)(milliseconds to wait=u32 20) -> ()  [unwired: 1 out]
                    }
                    n166 = call-poly <vilib>:"Mean.vi"("X"=w358) -> ("mean"=w356:dbl)  [unwired: 1 out]
                  }
                }
                n167 = Equal?(x=0, y=w290) -> (x = y?=w288:bool)
                n168 = Select(t=u32 3000, s=w288, f="milliseconds to wait") -> (s? t:f=w287:u32)
                n169 = Wait (ms)(milliseconds to wait=w287) -> ()  [unwired: 1 out]
                "#Итерации" <- w290
              }
              n170 = local write "Status:"("Построение характеристики TEC" ("Status:")) -> ()
              n171 = flat-sequence {
                tunnel: [T1."TRes_Check(Idle)" ("Case")] -> w273
                tunnel: w270 -> [w282]
                tunnel: [TRUE] -> w271
                tunnel: w268 -> [w280]
                tunnel: w268 -> [w278]
                tunnel: w267 -> [w277]
                frame #0 {
                  # "Построение харак-ки TEC\nи опциональная запись"
                  n172 = Bundle(w282, w280) -> (→"RES(I_TEC) Graph":cluster{dbl[], dbl[]})  [unwired: 1 in]
                  n173 = Bundle(w277, w278) -> (→"RES(U_TEC) Graph":cluster{dbl[], dbl[]})  [unwired: 1 in]
                  n174 = local write "Выполняется"(FALSE) -> ()
                }
              }
            }
            frame #3 {
              n175 = disable-structure shown="Disabled" {
                frame Disabled {
                  # "Переключение в режим Вольтметра"
                  n176 = local read "4070_Rele_source"() -> (w369:enum16{"S2_Ch0", "S1_Ch2"})
                  n177 = case shown="\"S2_Ch0\", Default" w369 {
                    tunnel: [0.0 0.0] -> w372
                    tunnel: ["0" "2"] -> w371
                    tunnel: [w373 w376] -> w370
                    frame "S2_Ch0", Default {
                      n178 = local read "Source_2_Vcc_out"() -> (w373:refnum<k15>)
                    }
                    frame "S1_Ch2" {
                      n179 = local read "Source_1_Vcc_out"() -> (w376:refnum<k15>)
                    }
                  }
                  n180 = call <instrlib>:"niDCPower Configure Voltage Level.vi"("voltage level"=w372, "channel name"=w371, "instrument handle"=w370) -> ()  [unwired: 7 in, 2 out]
                }
                frame Enabled {
                }
              }
              n181 = Wait (ms)(milliseconds to wait=u32 1000) -> ()  [unwired: 1 out]
              n182 = local write "ThRes_stabil"(TRUE) -> ()
            }
          }
        }
      }
      frame "TRes_Check(Idle)" {
        w387 = T4 7.5 items=["3 1/2"=3.5, "4 1/2"=4.5, "5 1/2"=5.5, "6 1/2"=6.5, "7 1/2"=7.5] ("Resolution in Digits")
        n183 = disable-structure shown="Disabled" {
          frame Disabled {
            w416 = T4 6.5 items=["3 1/2"=3.5, "4 1/2"=4.5, "5 1/2"=5.5, "6 1/2"=6.5, "7 1/2"=7.5] ("Resolution in Digits")
            n184 = local read "4070_address"() -> (w415:refnum<k15>)
            n185 = call-poly <instrlib>:"niDMM Config Measurement.vi"("Range"=-1.0 ("Configuration:Measurement Options:Max Frequency"), "Resolution in Digits"=w416, "Function"=niDMM_Function."2-wire Resistance" ("multimeter mode"), "instrument handle"=w415) -> ("instrument handle out"=w414:refnum<k15>)  [unwired: 6 in, 1 out]
            n186 = for {
              N: 3 -> [_]
              tunnel: w414 -> [w420]
              tunnel: [w419] -> w413 mode=indexing
              n187 = call <instrlib>:"niDMM Read.vi"("instrument handle"=w420) -> ("Measurement"=w419:dbl)  [unwired: 8 in, 2 out]
              n188 = Wait (ms)(milliseconds to wait=u32 50) -> ()  [unwired: 1 out]
            }
            n189 = call-poly <vilib>:"Mean.vi"("X"=w413) -> ("mean"=→"Сопротивление терморез-ра":dbl)  [unwired: 1 out]
          }
          frame Enabled {
          }
        }
        n190 = Wait (ms)(milliseconds to wait=u32 200) -> ()  [unwired: 1 out]
        n191 = local write "Status:"("IDLE" ("Status:")) -> ()
        n192 = local read "Использовать Офир?"() -> (w380:bool)
        n193 = case shown="True" w380 {
          frame False {
          }
          frame True {
            n194 = property on="Ophir_address" class="Ref (strict)"() -> ("Value"=w399:refnum<k7>)  [unwired: 2 in, 2 out]
            n195 = property on="hDevice" class="DigNum (strict)"() -> ("Value"=w398:i32)  [unwired: 2 in, 2 out]
            n196 = invoke class="ICoLMMeasurement" method="GetData"(reference=w399, "hDevice"=w398, "channel"=0) -> ("arrayValue"=w406:variant)  [unwired: 5 in, 7 out]
            n197 = Variant To Data(type=dbl[] [], Variant=w406) -> (data=w403:dbl[])  [unwired: 1 in, 1 out]
            n198 = Array Size(array=w403) -> (size(s)=w401:i32)
            n199 = Decrement(x=w401) -> (x-1=w400:i32)
            n200 = Index Array(array=w403, index=w400) -> (element=w402:dbl)
            n201 = Multiply(x=1000.0, y=w402) -> (x*y=→"Optical Power":dbl)
          }
        }
        n202 = local read "4071(1)_adress"() -> (w388:refnum<k15>)
        n203 = call-poly <instrlib>:"niDMM Config Measurement.vi"("Range"=-1.0 ("Configuration:Measurement Options:Max Frequency"), "Resolution in Digits"=w387, "Function"=niDMM_Function."DC Current" ("multimeter mode"), "instrument handle"=w388) -> ("instrument handle out"=w386:refnum<k15>)  [unwired: 6 in, 1 out]
        n204 = for {
          N: 5 -> [_]
          tunnel: w386 -> [w410]
          tunnel: [w408] -> w384 mode=indexing
          n205 = call <instrlib>:"niDMM Read.vi"("instrument handle"=w410) -> ("Measurement"=w408:dbl)  [unwired: 8 in, 2 out]
          n206 = Wait (ms)(milliseconds to wait=u32 50) -> ()  [unwired: 1 out]
        }
        n207 = call-poly <vilib>:"Mean.vi"("X"=w384) -> ("mean"=w383:dbl)  [unwired: 1 out]
        n208 = Absolute Value(x=w383) -> (abs(x)=w382:dbl)
        n209 = Multiply(x=w382, y=1000000.0) -> (x*y=w379:dbl)
        "I_pd, uA 2" <- w379
        n210 = local write "I_pd, uA"(w379) -> ()
        n211 = Select(t=T1."Quit" ("Case"), s="stop", f=T1."TRes_Check(Idle)" ("Case")) -> (s? t:f=w394:T1)
      }
      frame "Characteristics" {
        n212 = flat-sequence {
          tunnel: [w442] -> w432
          tunnel: [w446] -> w430
          tunnel: [w445] -> w428
          tunnel: [w444] -> w426
          tunnel: [w441] -> w424
          tunnel: [w438] -> w422
          tunnel: w432 -> [w698]
          tunnel: [w698] -> w431
          tunnel: w430 -> [w684]
          tunnel: [w684] -> w429
          tunnel: w428 -> [w700]
          tunnel: [w700] -> w427
          tunnel: w426 -> [w685]
          tunnel: [w685] -> w425
          tunnel: w424 -> [w699]
          tunnel: [w699] -> w423
          tunnel: w422 -> [w670]
          tunnel: [T1."TRes_Check(Idle)" ("Case")] -> w434
          tunnel: w431 -> [w702]
          tunnel: w429 -> [w719]
          tunnel: w427 -> [w718]
          tunnel: w425 -> [w716]
          tunnel: w423 -> [w713]
          frame #0 {
            n213 = local read "Отладка(F)/\n/Рабочий(T)"() -> (w435:bool)
            n214 = case shown="True" w435 {
              frame False {
              }
              frame True {
                n215 = while {
                  stop <- w437 stop-if-true
                  n216 = call "Save_dialogue_dose.vi"() -> ("output 1"=w436:dbl)  [unwired: 11 in]
                  n217 = Not Equal To 0?(x=w436) -> (x != 0?=w437:bool)
                  n218 = property on="Dose" class="DigNum (strict)"("Value"=w436) -> ()  [unwired: 2 in, 2 out]
                }
              }
            }
          }
          frame #1 {
            # "Хар-ки:\nI_LD (V);\nOphir(I_LD);\nI_PD(I_LD);\nRcheck(I_LD)"
            n219 = Subtract(x="Начальный ток, мА", y="Шаг, мА") -> (x-y=w447:dbl)
            n220 = for {
              N: "Кол-во точек" -> [_]
              shift-right: [w458] -> _
              shift-left: w447 -> [w460]
              tunnel: [w458] -> w442 mode=indexing
              tunnel: [w457] -> w446 mode=indexing
              tunnel: [w456] -> w445 mode=indexing
              tunnel: [w455] -> w444 mode=indexing
              tunnel: [w453] -> w441 mode=indexing
              shift-right: [w450] -> _
              shift-left: "Start voltage_LD" -> [w451]
              tunnel: [w449] -> w438
              i -> [w454]
              # "ExtPD"
              # "FV"
              # "I_PD"
              # "I_LD"
              # "Ophir"
              n221 = property on="Шаг, мА" class="DigNum (strict)"() -> ("Value"=w452:dbl)  [unwired: 2 in, 2 out]
              n222 = Add(x=w460, y=w452) -> (x+y=w459:dbl)
              n223 = stacked-sequence {
                tunnel: w459 -> [_ w482 _ _ _ _ _ _ _ _]
                tunnel: [_ w477 _ _ _ _ _ _ _ _] -> w458
                tunnel: [_ _ _ _ _ w545 _ _ _ _] -> w457
                tunnel: [_ _ _ _ _ _ w562 _ _ _] -> w456
                tunnel: [_ _ _ _ w535 _ _ _ _ _] -> w455
                tunnel: w454 -> [_ _ _ _ _ _ _ _ w598 _]
                tunnel: [_ _ _ _ _ _ _ w575 _ _] -> w453
                tunnel: w451 -> [_ w474 _ _ _ _ _ _ _ _]
                tunnel: [_ w473 _ _ _ _ _ _ _ _] -> w450
                tunnel: [_ _ _ _ _ _ _ _ _ w667] -> w449
                frame #0 {
                  n224 = disable-structure shown="Disabled" {
                    frame Disabled {
                      n225 = stacked-sequence {
                        frame #0 {
                          w461 = FALSE
                          # "Отключение стабилизации"
                          n226 = while {
                            tunnel: w461 -> [_]
                            stop <- w462 stop-if-true
                            n227 = local read "NoStab"() -> (w462:bool)
                          }
                          n228 = local write "ThRes_stabil"(w461) -> ()
                        }
                        frame #1 {
                          # "Переключение в режим Вольтметра"
                          n229 = local read "4070_Rele_source"() -> (w463:enum16{"S2_Ch0", "S1_Ch2"})
                          n230 = case shown="\"S2_Ch0\", Default" w463 {
                            tunnel: [0.0 0.0] -> w466
                            tunnel: ["0" "2"] -> w465
                            tunnel: [w467 w470] -> w464
                            frame "S2_Ch0", Default {
                              n231 = local read "Source_2_Vcc_out"() -> (w467:refnum<k15>)
                            }
                            frame "S1_Ch2" {
                              n232 = local read "Source_1_Vcc_out"() -> (w470:refnum<k15>)
                            }
                          }
                          n233 = call <instrlib>:"niDCPower Configure Voltage Level.vi"("voltage level"=w466, "channel name"=w465, "instrument handle"=w464) -> ()  [unwired: 7 in, 2 out]
                        }
                      }
                    }
                    frame Enabled {
                    }
                  }
                }
                frame #1 {
                  # "Подстройка тока\nлазерного диода"
                  n234 = local read "Source_1_Vcc_out"() -> (w483:refnum<k15>)
                  n235 = disable-structure shown="Enabled" {
                    disable-tunnel: "the lower limit for the voltage_LD" -> [w499 w505]
                    disable-tunnel: w474 -> [w498 w506]
                    disable-tunnel: "the upper limit for the voltage_LD" -> [w497 w507]
                    disable-tunnel: w483 -> [w496 w504]
                    disable-tunnel: w482 -> [w495 w503]
                    disable-tunnel: "Res_LD" -> [w494 w502]
                    disable-tunnel: "0" -> [w493 w500]
                    disable-tunnel: "accuracy_LD" -> [w492 w510]
                    disable-tunnel: [w491 w509] -> w473
                    disable-tunnel: [w489 w508] -> w478
                    disable-tunnel: [w488 w501] -> w477
                    frame Disabled {
                      n236 = local read "4070_address"() -> (w490:refnum<k15>)
                      n237 = call "Set input current_ChAmmeter.vi"("the lower limit for the voltage"=w499, "accuracy (input)"=w492, "4070_address"=w490, "Start voltage"=w498, "the upper limit for the voltage"=w497, "instrument handle"=w496, "the optimum current(input)"=w495, "res(input)"=w494, "channel name"=w493) -> ("accommodated voltage (out)"=w491:dbl, "current value, mA"=w488:dbl, "the voltage drop across the resistor"=w489:dbl)  [unwired: 3 in, 1 out]
                    }
                    frame Enabled {
                      n238 = call "Set input current_ChSource.vi"("channel name"=w500, "res(input)"=w502, "the optimum current(input)"=w503, "accuracy (input)"=w510, "instrument handle"=w504, "the upper limit for the voltage"=w507, "Start voltage"=w506, "the lower limit for the voltage"=w505) -> ("current value, mA"=w501:dbl, "the voltage drop across the resistor"=w508:dbl, "accommodated voltage (out)"=w509:dbl)  [unwired: 1 out]
                    }
                  }
                  "Подстроенный ток, mA" <- w477
                  "accommodated voltage (out)" <- w473
                  "Volt_onRes" <- w478
                  n239 = local write "Status:"("Подстройка тока LD" ("Status:")) -> ()
                  n240 = Wait (ms)(milliseconds to wait=u32 100) -> ()  [unwired: 1 out]
                  n241 = Greater Or Equal?(x=w477, y=49.0) -> (x >= y?=→"Boolean":bool)
                }
                frame #2 {
                  # "and stab"
                  # "Resistance check"
                  n242 = flat-sequence {
                    frame #0 {
                      n243 = disable-structure shown="Disabled" {
                        frame Disabled {
                          # "Режим Омметра"
                          n244 = case shown="\"S2_Ch0\", Default" "4070_Rele_source" {
                            tunnel: [5.0 -5.0] -> w514
                            tunnel: ["0" "2"] -> w513
                            tunnel: [w516 w519] -> w512
                            frame "S2_Ch0", Default {
                              n245 = local read "Source_2_Vcc_out"() -> (w516:refnum<k15>)
                            }
                            frame "S1_Ch2" {
                              n246 = local read "Source_1_Vcc_out"() -> (w519:refnum<k15>)
                            }
                          }
                          n247 = call <instrlib>:"niDCPower Configure Voltage Level.vi"("voltage level"=w514, "channel name"=w513, "instrument handle"=w512) -> ()  [unwired: 7 in, 2 out]
                        }
                        frame Enabled {
                        }
                      }
                    }
                    frame #1 {
                      n248 = Wait (ms)(milliseconds to wait=u32 1000) -> ()  [unwired: 1 out]
                      "Num_hits" <- u64 0 ("Num_hits")
                    }
                    frame #2 {
                      n249 = local write "ThRes_stabil"(TRUE) -> ()
                    }
                    frame #3 {
                      n250 = local write "Count_hits?"(TRUE ("Acq_allow?")) -> ()
                      n251 = Wait (ms)(milliseconds to wait="tstab между точками, мс") -> ()  [unwired: 1 out]
                    }
                  }
                  n252 = local write "Status:"("Проверка и стабилизация сопротивления" ("Status:")) -> ()
                }
                frame #3 {
                  n253 = while {
                    tunnel: [u64 0] -> w528
                    tunnel: [FALSE ("Acq_allow?")] -> w527
                    stop <- w531 stop-if-true
                    n254 = local read "Num_hits"() -> (w533:u64)
                    n255 = Greater Or Equal?(x=w533, y="Num_hits_req") -> (x >= y?=w531:bool)
                  }
                  n256 = local write "Count_hits?"(w527) -> ()
                  n257 = local write "Num_hits"(w528) -> ()
                }
                frame #4 {
                  # "Forward\nVoltage\nmeasurement"
                  n258 = local read "Source_1_Vcc_out"() -> (w541:refnum<k15>)
                  n259 = local read "Volt_onRes"() -> (w534:dbl)
                  n260 = call <instrlib>:"niDCPower Measure Multiple.vi"("channel name"="0", "instrument handle"=w541) -> ("voltage measurements"=w539:dbl[])  [unwired: 6 in, 3 out]
                  n261 = Index Array(array=w539) -> (element=w537:dbl)  [unwired: 1 in]
                  n262 = Absolute Value(x=w534) -> (abs(x)=w536:dbl)
                  n263 = Absolute Value(x=w537) -> (abs(x)=w538:dbl)
                  n264 = Subtract(x=w538, y=w536) -> (x-y=w535:dbl)
                  "Forward Voltage, V" <- w535
                  n265 = local write "Status:"("Измерение прямого напряжения" ("Status:")) -> ()
                  n266 = Wait (ms)(milliseconds to wait=u32 100) -> ()  [unwired: 1 out]
                }
                frame #5 {
                  n267 = local read "Использовать Офир?"() -> (w544:bool)
                  n268 = case shown="True" w544 {
                    tunnel: [_ w547] -> w545
                    frame False {
                    }
                    frame True {
                      # "Ophir\nmeasurement"
                      n269 = property on="Ophir_address" class="Ref (strict)"() -> ("Value"=w549:refnum<k7>)  [unwired: 2 in, 2 out]
                      n270 = property on="hDevice" class="DigNum (strict)"() -> ("Value"=w548:i32)  [unwired: 2 in, 2 out]
                      n271 = invoke class="ICoLMMeasurement" method="GetData"(reference=w549, "hDevice"=w548, "channel"=0) -> ("arrayValue"=w556:variant)  [unwired: 5 in, 7 out]
                      n272 = Variant To Data(type=dbl[] [], Variant=w556) -> (data=w553:dbl[])  [unwired: 1 in, 1 out]
                      n273 = Wait (ms)(milliseconds to wait=u32 200) -> ()  [unwired: 1 out]
                      n274 = Array Size(array=w553) -> (size(s)=w551:i32)
                      n275 = Decrement(x=w551) -> (x-1=w550:i32)
                      n276 = Index Array(array=w553, index=w550) -> (element=w552:dbl)
                      n277 = Multiply(x=1000.0, y=w552) -> (x*y=w547:dbl)
                      "Ophir, mW" <- w547
                      n278 = local write "Optical Power"(w547) -> ()
                    }
                  }
                  n279 = local write "Status:"("Измерен. оптич. мощности" ("Status:")) -> ()
                }
                frame #6 {
                  w565 = T4 7.5 items=["3 1/2"=3.5, "4 1/2"=4.5, "5 1/2"=5.5, "6 1/2"=6.5, "7 1/2"=7.5] ("Resolution in Digits")
                  # "Inside I_PD\nmeasurements"
                  n280 = local read "4071(1)_adress"() -> (w566:refnum<k15>)
                  n281 = call-poly <instrlib>:"niDMM Config Measurement.vi"("Range"=-1.0 ("Configuration:Measurement Options:Max Frequency"), "Resolution in Digits"=w565, "Function"=niDMM_Function."DC Current" ("multimeter mode"), "instrument handle"=w566) -> ("instrument handle out"=w564:refnum<k15>)  [unwired: 6 in, 1 out]
                  n282 = for {
                    N: 5 -> [_]
                    tunnel: w564 -> [w573]
                    tunnel: [w570] -> w559 mode=indexing
                    n283 = call <instrlib>:"niDMM Read.vi"("instrument handle"=w573) -> ("Measurement"=w571:dbl)  [unwired: 8 in, 2 out]
                    n284 = Absolute Value(x=w571) -> (abs(x)=w570:dbl)
                    n285 = Wait (ms)(milliseconds to wait=u32 50) -> ()  [unwired: 1 out]
                  }
                  n286 = local write "Status:"("I_PD встроенного фотодиода" ("Status:")) -> ()
                  n287 = call-poly <vilib>:"Mean.vi"("X"=w559) -> ("mean"=w560:dbl)  [unwired: 1 out]
                  n288 = Multiply(x=w560, y=1000000.0) -> (x*y=w562:dbl)
                  "I_pd, uA" <- w562
                }
                frame #7 {
                  # "EXTERNAL I_PD\nmeasurements"
                  n289 = disable-structure shown="Enabled" {
                    disable-tunnel: [w578 w593] -> w575
                    disable-tunnel: [_ w593] -> w574
                    frame Disabled {
                      w585 = T4 6.5 items=["3 1/2"=3.5, "4 1/2"=4.5, "5 1/2"=5.5, "6 1/2"=6.5, "7 1/2"=7.5] ("Resolution in Digits")
                      n290 = local read "4071(2)_adress"() -> (w586:refnum<k15>)
                      n291 = call-poly <instrlib>:"niDMM Config Measurement.vi"("Range"=-1.0 ("Configuration:Measurement Options:Max Frequency"), "Resolution in Digits"=w585, "Function"=niDMM_Function."DC Current" ("multimeter mode"), "instrument handle"=w586) -> ("instrument handle out"=w584:refnum<k15>)  [unwired: 6 in, 1 out]
                      n292 = for {
                        N: 5 -> [_]
                        tunnel: w584 -> [w591]
                        tunnel: [w589] -> w582 mode=indexing
                        n293 = call <instrlib>:"niDMM Read.vi"("instrument handle"=w591) -> ("Measurement"=w589:dbl)  [unwired: 8 in, 2 out]
                        n294 = Wait (ms)(milliseconds to wait=u32 50) -> ()  [unwired: 1 out]
                      }
                      n295 = call-poly <vilib>:"Mean.vi"("X"=w582) -> ("mean"=w581:dbl)  [unwired: 1 out]
                      n296 = Absolute Value(x=w581) -> (abs(x)=w580:dbl)
                      n297 = Multiply(x=w580, y=1000.0) -> (x*y=w578:dbl)
                    }
                    frame Enabled {
                      n298 = local read "Source_2_Vcc_out"() -> (w597:refnum<k15>)
                      n299 = call <instrlib>:"niDCPower Measure Multiple.vi"("channel name"="1", "instrument handle"=w597) -> ("current measurements"=w595:dbl[])  [unwired: 6 in, 3 out]
                      n300 = Index Array(array=w595) -> (element=w592:dbl)  [unwired: 1 in]
                      n301 = Multiply(x=w592, y=1000.0) -> (x*y=w593:dbl)
                    }
                  }
                  "IPD(ext), mA" <- w574
                  n302 = local write "Status:"("I_PD внешнего фотодиода" ("Status:")) -> ()
                  n303 = Wait (ms)(milliseconds to wait=u32 200) -> ()  [unwired: 1 out]
                }
                frame #8 {
                  n304 = local read "Отладка(F)/\n/Рабочий(T)"() -> (w599:bool)
                  n305 = case shown="True" w599 {
                    tunnel: w598 -> [_ w619]
                    frame False {
                    }
                    frame True {
                      w609 = i16 3 ("width (-)")
                      w610 = i16 3 ("width (-)")
                      w612 = i16 3 ("width (-)")
                      w615 = i16 3 ("width (-)")
                      w618 = i16 3 ("width (-)")
                      # "Внешний ФД"
                      # "Офир"
                      n306 = local read "IPD(ext), mA"() -> (w603:dbl)
                      n307 = local read "Ophir, mW"() -> (w602:dbl)
                      n308 = local read "Forward Voltage, V"() -> (w614:dbl)
                      n309 = local read "Подстроенный ток, mA"() -> (w617:dbl)
                      n310 = local read "I_pd, uA"() -> (w611:dbl)
                      n311 = Equal To 0?(x=w619) -> (x = 0?=w607:bool)
                      n312 = Number To Fractional String(number=w617, width (-)=w618, precision (6)=w618) -> (F-format string=w616:string)  [unwired: 1 in]
                      n313 = Number To Fractional String(number=w614, width (-)=w615, precision (6)=w615) -> (F-format string=w613:string)  [unwired: 1 in]
                      n314 = Number To Fractional String(number=w603, width (-)=w612, precision (6)=w612) -> (F-format string=w604:string)  [unwired: 1 in]
                      n315 = Number To Fractional String(number=w611, width (-)=w610, precision (6)=w610) -> (F-format string=w605:string)  [unwired: 1 in]
                      n316 = Number To Fractional String(number=w602, width (-)=w609, precision (6)=w609) -> (F-format string=w606:string)  [unwired: 1 in]
                      n317 = case shown="True" w607 {
                        tunnel: [w620 w623] -> w601
                        tunnel: [w620 w622] -> w608
                        tunnel: [w620 w621] -> w600
                        frame False {
                          w620 = "" ("date/time string")
                        }
                        frame True {
                          n318 = stacked-sequence {
                            tunnel: [w627 _] -> w623
                            tunnel: [w624 _] -> w622
                            tunnel: [_ w630] -> w621
                            frame #0 {
                              w626 = i16 0 ("width (-)")
                              n319 = Get Date/Time In Seconds() -> (seconds since 1Jan1904=w629:timestamp)
                              n320 = Format Date/Time String(time format string (%c)="%d  %H:%M:%S", seconds (now)=w629) -> (date/time string=w627:string)  [unwired: 1 in]
                              n321 = Number To Fractional String(number="Dose", width (-)=w626, precision (6)=w626) -> (F-format string=w624:string)  [unwired: 1 in]
                            }
                            frame #1 {
                              n322 = local read "Использовать Офир?"() -> (w631:bool)
                              n323 = Select(t="С Офиром", s=w631, f="Без Офира") -> (s? t:f=w630:string)
                            }
                          }
                        }
                      }
                      n324 = stacked-sequence {
                        tunnel: w601 -> [w641 w649 w657 _ w665]
                        tunnel: w608 -> [w639 w647 w655 _ w663]
                        tunnel: w616 -> [w638 w646 w654 _ w660]
                        tunnel: w613 -> [w636 _ _ _ _]
                        tunnel: w606 -> [_ w645 _ _ _]
                        tunnel: w605 -> [_ _ w652 _ _]
                        tunnel: w604 -> [_ _ _ _ w662]
                        tunnel: w600 -> [w634 w642 w650 _ w658]
                        frame #0 {
                          w637 = "\t"
                          n325 = local read "V2(Ild)_Log_address"() -> (w640:refnum<file>)
                          n326 = Format Into String(initial string=w640, w641, w637, w634, w637, w639, w637, w638, w637, w636, "\r\n") -> ()  [unwired: 2 in, 2 out]
                        }
                        frame #1 {
                          w644 = "\t"
                          n327 = local read "Op(Ild)_Log_address"() -> (w648:refnum<file>)
                          n328 = Format Into String(initial string=w648, w649, w644, w642, w644, w647, w644, w646, w644, w645, "\r\n") -> ()  [unwired: 2 in, 2 out]
                        }
                        frame #2 {
                          w653 = "\t"
                          n329 = local read "Ipd(Ild)_Monitor_Log_address"() -> (w656:refnum<file>)
                          n330 = Format Into String(initial string=w656, w657, w653, w650, w653, w655, w653, w654, w653, w652, "\r\n") -> ()  [unwired: 2 in, 2 out]
                        }
                        frame #3 {
                        }
                        frame #4 {
                          w661 = "\t"
                          n331 = local read "Ipd(Ild)_External_Log_address"() -> (w664:refnum<file>)
                          n332 = Format Into String(initial string=w664, w665, w661, w658, w661, w663, w661, w660, w661, w662, "\r\n") -> ()  [unwired: 2 in, 2 out]
                        }
                      }
                    }
                  }
                }
                frame #9 {
                  n333 = local read "Использовать Офир?"() -> (w668:bool)
                  n334 = Select(t="С Офиром", s=w668, f="Без Офира") -> (s? t:f=w667:string)
                }
              }
            }
          }
          frame #2 {
            w673 = i16 0 ("width (-)")
            w681 = i16 3 ("width (-)")
            w687 = i16 3 ("width (-)")
            w689 = i16 3 ("width (-)")
            w692 = i16 3 ("width (-)")
            w679 = "\t"
            w696 = i16 3 ("width (-)")
            # "Рабочее напряжение"
            n335 = Get Date/Time In Seconds() -> ()  [unwired: 1 out]
            n336 = local read "Ophir, mW"() -> (w686:dbl)
            n337 = call "Find_ThresholdOphir_F4.vi"("Threshold Ophir"=5.0, "Current array"=w685, "Ophir array"=w684) -> ("Threshold Current"=w682:dbl)  [unwired: 8 in]
            n338 = call "Find_ThresholdOphir_F4.vi"("Threshold Ophir"=1.0, "Current array"=w698, "Ophir array"=w684) -> ("Threshold Current"=w695:dbl)  [unwired: 8 in]
            "Пороговый ток" <- w695
            n339 = local read "I_pd, uA"() -> (w680:dbl)
            n340 = local read "Подстроенный ток, mA"() -> (w691:dbl)
            n341 = Format Date/Time String(time format string (%c)="%d  %H:%M:%S") -> (date/time string=w674:string)  [unwired: 2 in]
            n342 = Number To Fractional String(number=w682, width (-)=w689, precision (6)=w689) -> (F-format string=w688:string)  [unwired: 1 in]
            n343 = Number To Fractional String(number=w695, width (-)=w696, precision (6)=w696) -> (F-format string=w693:string)  [unwired: 1 in]
            n344 = Number To Fractional String(number=w680, width (-)=w681, precision (6)=w681) -> (F-format string=w677:string)  [unwired: 1 in]
            n345 = Number To Fractional String(number=w686, width (-)=w687, precision (6)=w687) -> (F-format string=w676:string)  [unwired: 1 in]
            n346 = local read "Dose"() -> (w672:i32)
            n347 = Number To Fractional String(number=w691, width (-)=w692, precision (6)=w692) -> (F-format string=w690:string)  [unwired: 1 in]
            n348 = local read "Param_Log_address"() -> (w694:refnum<file>)
            n349 = Number To Fractional String(number=w672, width (-)=w673, precision (6)=w673) -> (F-format string=w671:string)  [unwired: 1 in]
            n350 = Format Into String(initial string=w694, w674, w679, w670, w679, w671, w679, w693, w679, w690, w679, w688, w679, w677, w679, w676, "\r\n") -> ()  [unwired: 2 in, 2 out]
          }
          frame #3 {
            n351 = local read "Source_1_Vcc_out"() -> (w711:refnum<k15>)
            n352 = local read "Подстроенное напряжение\nстабилизации"() -> (w708:dbl)
            n353 = case shown="True" "Оставить в раб.\nрежиме" {
              tunnel: [0.0 ("voltage level") w724] -> w710
              frame False {
              }
              frame True {
                n354 = local read "accommodated voltage (out)"() -> (w724:dbl)
              }
            }
            n355 = local read "Source_1_Vcc_out"() -> (w707:refnum<k15>)
            n356 = Bundle(w702, w719) -> (→"OP(I_LD) Graph":cluster{dbl[], dbl[]})  [unwired: 1 in]
            n357 = Bundle(w702, w718) -> (→"I_PD(I_LD) Graph":cluster{dbl[], dbl[]})  [unwired: 1 in]
            n358 = Bundle(w702, w716) -> (→"V2(I_LD) Graph":cluster{dbl[], dbl[]})  [unwired: 1 in]
            n359 = Bundle(w702, w713) -> (→"I_PD_Ext(I_LD) Graph":cluster{dbl[], dbl[]})  [unwired: 1 in]
            n360 = Add(x=w708, y=0.2) -> (x+y=w703:dbl)
            n361 = local write "Выполняется"(FALSE) -> ()
            n362 = Multiply(x=w703, y=-1.0) -> (x*y=w704:dbl)
            n363 = call <instrlib>:"niDCPower Configure Voltage Level.vi"("voltage level"=w704, "channel name"="2", "instrument handle"=w707) -> ()  [unwired: 7 in, 2 out]
            n364 = call <instrlib>:"niDCPower Configure Voltage Level.vi"("voltage level"=w710, "channel name"="0", "instrument handle"=w711) -> ()  [unwired: 7 in, 2 out]
          }
        }
        n365 = local write "Boolean 2"(FALSE) -> ()
      }
      frame "Bias" {
        n366 = local write "Boolean 2"(FALSE) -> ()
        n367 = stacked-sequence {
          tunnel: [_ _ _ T1."TRes_Check(Idle)" ("Case")] -> w726
          frame #0 {
            n368 = disable-structure shown="Disabled" {
              frame Disabled {
                w728 = FALSE
                n369 = while {
                  tunnel: w728 -> [_]
                  stop <- w729 stop-if-true
                  n370 = local read "NoStab"() -> (w729:bool)
                }
                n371 = local write "ThRes_stabil"(w728) -> ()
              }
              frame Enabled {
              }
            }
            n372 = local write "Num_hits"(0) -> ()
          }
          frame #1 {
            n373 = disable-structure shown="Disabled" {
              frame Disabled {
                # "Переключение в режим Вольтметра"
                n374 = local read "4070_Rele_source"() -> (w730:enum16{"S2_Ch0", "S1_Ch2"})
                n375 = case shown="\"S2_Ch0\", Default" w730 {
                  tunnel: [0.0 0.0] -> w733
                  tunnel: ["0" "2"] -> w732
                  tunnel: [w734 w737] -> w731
                  frame "S2_Ch0", Default {
                    n376 = local read "Source_2_Vcc_out"() -> (w734:refnum<k15>)
                  }
                  frame "S1_Ch2" {
                    n377 = local read "Source_1_Vcc_out"() -> (w737:refnum<k15>)
                  }
                }
                n378 = call <instrlib>:"niDCPower Configure Voltage Level.vi"("voltage level"=w733, "channel name"=w732, "instrument handle"=w731) -> ()  [unwired: 7 in, 2 out]
              }
              frame Enabled {
              }
            }
          }
          frame #2 {
            n379 = local read "the upper limit for the voltage_LD"() -> (w754:dbl)
            n380 = local read "the lower limit for the voltage_LD"() -> (w756:dbl)
            n381 = local read "Source_1_Vcc_out"() -> (w753:refnum<k15>)
            n382 = local read "Start voltage_LD"() -> (w755:dbl)
            n383 = local read "accuracy_LD"() -> (w750:dbl)
            n384 = local read "Res_LD"() -> (w752:dbl)
            n385 = disable-structure shown="Enabled" {
              disable-tunnel: "Desirable Operating current, mA" -> [w769 w775]
              disable-tunnel: [w768 w776] -> w757
              disable-tunnel: w756 -> [w767 w779]
              disable-tunnel: w755 -> [w766 w770]
              disable-tunnel: w754 -> [w765 w771]
              disable-tunnel: w753 -> [w764 w772]
              disable-tunnel: w752 -> [w763 w774]
              disable-tunnel: "0" ("channel name") -> [w762 w773]
              disable-tunnel: w750 -> [w761 w778]
              disable-tunnel: [w760 w777] -> w749
              frame Disabled {
                n386 = local read "4070_address"() -> (w759:refnum<k15>)
                n387 = call "Set input current_ChAmmeter.vi"("the lower limit for the voltage"=w767, "accuracy (input)"=w761, "4070_address"=w759, "Start voltage"=w766, "the upper limit for the voltage"=w765, "instrument handle"=w764, "the optimum current(input)"=w769, "res(input)"=w763, "channel name"=w762) -> ("accommodated voltage (out)"=w760:dbl, "current value, mA"=w768:dbl)  [unwired: 3 in, 2 out]
              }
              frame Enabled {
                n388 = call "Set input current_ChSource.vi"("channel name"=w773, "res(input)"=w774, "the optimum current(input)"=w775, "accuracy (input)"=w778, "instrument handle"=w772, "the upper limit for the voltage"=w771, "Start voltage"=w770, "the lower limit for the voltage"=w779) -> ("current value, mA"=w776:dbl, "accommodated voltage (out)"=w777:dbl)  [unwired: 2 out]
              }
            }
            "Operating Current, mA" <- w757
            n389 = local read "+ V TEC для новой точки"() -> (w744:dbl)
            n390 = local read "Подстроенное напряжение\nстабилизации"() -> (w742:dbl)
            n391 = local read "Source_1_Vcc_out"() -> (w748:refnum<k15>)
            n392 = local write "accommodated voltage (out)"(w749) -> ()
            n393 = Multiply(x=w744, y=2.0) -> (x*y=w741:dbl)
            n394 = Add(x=w741, y=w742) -> (x+y=w740:dbl)
            n395 = Multiply(x=w740, y=-1.0) -> (x*y=w745:dbl)
            n396 = call <instrlib>:"niDCPower Configure Voltage Level.vi"("voltage level"=w745, "channel name"="2", "instrument handle"=w748) -> ()  [unwired: 7 in, 2 out]
          }
          frame #3 {
            n397 = disable-structure shown="Enabled" {
              frame Disabled {
                # "Переключение в режим Омметра"
                n398 = local read "4070_Rele_source"() -> (w786:enum16{"S2_Ch0", "S1_Ch2"})
                n399 = case shown="\"S2_Ch0\", Default" w786 {
                  tunnel: [5.0 -5.0] -> w785
                  tunnel: ["0" "2"] -> w784
                  tunnel: [w787 w790] -> w783
                  frame "S2_Ch0", Default {
                    n400 = local read "Source_2_Vcc_out"() -> (w787:refnum<k15>)
                  }
                  frame "S1_Ch2" {
                    n401 = local read "Source_1_Vcc_out"() -> (w790:refnum<k15>)
                  }
                }
                n402 = call <instrlib>:"niDCPower Configure Voltage Level.vi"("voltage level"=w785, "channel name"=w784, "instrument handle"=w783) -> ()  [unwired: 7 in, 2 out]
              }
              frame Enabled {
              }
            }
            n403 = local write "Выполняется"(FALSE) -> ()
            n404 = local write "ThRes_stabil"(TRUE) -> ()
          }
        }
      }
      frame "Quit" {
        w794 = FALSE
        n405 = local write "Status:"("Выход" ("Status:")) -> ()
        n406 = local write "Num_hits"(u64 0 ("Num_hits")) -> ()
        n407 = local write "stop"(w794) -> ()
        n408 = local write "Power Enable"(w794) -> ()
        n409 = local write "Прервать"(w794) -> ()
        n410 = local write "Count_hits?"(w794) -> ()
      }
    }
  }
  n411 = while {
    shift-right: [w803] -> _
    shift-left: w1 -> [w799]
    tunnel: w3 -> [w802]
    stop <- FALSE stop-if-true
    n412 = local read "ThRes_stabil"() -> (w804:bool)
    n413 = Select(t="Напряжение Пельтье", s="В ручную", f=w799) -> (s? t:f=w798:dbl)
    n414 = case shown="True" w804 {
      tunnel: [w807 w815] -> w803
      tunnel: w798 -> [_ w821]
      tunnel: w802 -> [_ _]
      frame False {
        n415 = local read "Подстроенное напряжение\nстабилизации"() -> (w806:dbl)
        n416 = local read "Source_1_Vcc_out"() -> (w811:refnum<k15>)
        n417 = local write "NoStab"(TRUE) -> ()
        n418 = Add(x="+ V TEC для новой точки", y=w806) -> (x+y=w807:dbl)
        n419 = Multiply(x=w807, y=-1.0) -> (x*y=w808:dbl)
        n420 = call <instrlib>:"niDCPower Configure Voltage Level.vi"("voltage level"=w808, "channel name"="2", "instrument handle"=w811) -> ()  [unwired: 7 in, 2 out]
      }
      frame True {
        w817 = T4 6.5 items=["3 1/2"=3.5, "4 1/2"=4.5, "5 1/2"=5.5, "6 1/2"=6.5, "7 1/2"=7.5] ("Resolution in Digits")
        n421 = local read "TEC_Source"() -> (w824:enum16{"S1_Ch2", "S2_Ch0", "S3_Ch1"})
        n422 = local read "the upper limit for the voltage"() -> (w822:dbl)
        n423 = local read "the lower limit for the voltage"() -> (w823:dbl)
        n424 = local read "4070_address"() -> (w816:refnum<k15>)
        n425 = case shown="\"S1_Ch2\", Default" w824 {
          tunnel: [w829 w831 w833] -> w826
          tunnel: ["2" "0" "1"] -> w825
          frame "S1_Ch2", Default {
            n426 = local read "Source_1_Vcc_out"() -> (w829:refnum<k15>)
          }
          frame "S2_Ch0" {
            n427 = local read "Source_2_Vcc_out"() -> (w831:refnum<k15>)
          }
          frame "S3_Ch1" {
            n428 = local read "Source_3_Vcc_out"() -> (w833:refnum<k15>)
          }
        }
        n429 = call-poly <instrlib>:"niDMM Config Measurement.vi"("Range"=-1.0 ("Configuration:Measurement Options:Max Frequency"), "Resolution in Digits"=w817, "Function"=niDMM_Function."2-wire Resistance" ("multimeter mode"), "instrument handle"=w816) -> ("instrument handle out"=w814:refnum<k15>)  [unwired: 6 in, 1 out]
        n430 = while {
          tunnel: w825 -> [w841]
          tunnel: w826 -> [w842]
          tunnel: w814 -> [w840]
          shift-right: [w839] -> w815
          shift-left: w821 -> [w843]
          tunnel: [w837] -> w827
          tunnel: w823 -> [w835]
          tunnel: w822 -> [w834]
          i -> [w847]
          stop <- w848 stop-if-true
          n431 = local read "Optimum ThRes"() -> (w836:dbl)
          n432 = Greater Or Equal?(x=w843, y=w835) -> (x >= y?=w846:bool)
          n433 = Less Or Equal?(x=w843, y=w834) -> (x <= y?=w845:bool)
          n434 = And(x=w846, y=w845) -> (x .and. y?=w844:bool)
          n435 = case shown="True" w844 {
            tunnel: w843 -> [_ w856]
            tunnel: w842 -> [_ w858]
            tunnel: w841 -> [_ w857]
            tunnel: w836 -> [_ w854]
            tunnel: w840 -> [_ w855]
            tunnel: [0.5 w853] -> w839
            tunnel: [_ w852] -> w838
            frame False {
            }
            frame True {
              n436 = stacked-sequence {
                seq-local: [w859 _ _] -> [_ _ w886]
                seq-local: [_ w866 _] -> [_ _ w876]
                tunnel: w858 -> [w864 _ _]
                tunnel: w857 -> [w863 _ _]
                tunnel: w856 -> [w859 _ _]
                tunnel: w855 -> [_ w865 _]
                tunnel: w854 -> [_ _ w879]
                tunnel: [_ _ w885] -> w853
                tunnel: [_ _ w884] -> w852
                frame #0 {
                  n437 = Multiply(x=w859, y=-1.0) -> (x*y=w860:dbl)
                  n438 = call <instrlib>:"niDCPower Configure Voltage Level.vi"("voltage level"=w860, "channel name"=w863, "instrument handle"=w864) -> ()  [unwired: 7 in, 2 out]
                  n439 = Wait (ms)(milliseconds to wait="Source-Ohm w8") -> ()  [unwired: 1 out]
                }
                frame #1 {
                  n440 = for {
                    N: 5 -> [_]
                    tunnel: w865 -> [w871]
                    tunnel: [w870] -> w867 mode=indexing
                    n441 = call <instrlib>:"niDMM Read.vi"("instrument handle"=w871) -> ("Measurement"=w870:dbl)  [unwired: 8 in, 2 out]
                    n442 = Wait (ms)(milliseconds to wait=u32 10) -> ()  [unwired: 1 out]
                  }
                  n443 = call-poly <vilib>:"Mean.vi"("X"=w867) -> ("mean"=w866:dbl)  [unwired: 1 out]
                  "thRes_adj" <- w866
                  n444 = local write "Сопротивление терморез-ра"(w866) -> ()
                }
                frame #2 {
                  # "Показания Терморезистора"
                  n445 = local read "Точность ThRes"() -> (w883:dbl)
                  n446 = Subtract(x=w879, y=w883) -> (x-y=w889:dbl)
                  n447 = Add(x=w879, y=w883) -> (x+y=w890:dbl)
                  n448 = Greater Or Equal?(x=w876, y=w889) -> (x >= y?=w891:bool)
                  n449 = Less Or Equal?(x=w876, y=w890) -> (x <= y?=w888:bool)
                  n450 = Subtract(x=w879, y="Coeff_thr") -> (x-y=w877:dbl)
                  n451 = Add(x="Coeff_thr", y=w879) -> (x+y=w875:dbl)
                  n452 = And(x=w891, y=w888) -> (x .and. y?=w887:bool)
                  n453 = Greater Or Equal?(x=w876, y=w877) -> (x >= y?=w874:bool)
                  n454 = Less Or Equal?(x=w876, y=w875) -> (x <= y?=w873:bool)
                  n455 = And(x=w874, y=w873) -> (x .and. y?=w872:bool)
                  n456 = Select(t="Coeff_High", s=w872, f="Coeff_low") -> (s? t:f=w880:dbl)
                  n457 = case shown="True" w887 {
                    tunnel: [w893 w908] -> w885
                    tunnel: w886 -> [w895 w909]
                    tunnel: [_ TRUE] -> w884
                    tunnel: w876 -> [w896 w915]
                    tunnel: w879 -> [w897 _]
                    tunnel: w880 -> [w892 _]
                    frame False {
                      n458 = Subtract(x=w897, y=w896) -> (x-y=w898:dbl)
                      "Разница ThRes" <- w898
                      n459 = Divide(x=w898, y=w892) -> (x/y=w894:dbl)
                      "+Voltage\nrequired" <- w894
                      n460 = Add(x=w894, y=w895) -> (x+y=w893:dbl)
                    }
                    frame True {
                      # "тут был \"выполняется\" не"
                      n461 = local read "Boolean 2"() -> (w899:bool)
                      n462 = local read "Num_hits"() -> (w913:u64)
                      n463 = case shown="False" "Count_hits?" {
                        frame False {
                          n464 = local read "Num_hits"() -> (w917:u64)
                          n465 = Increment(x=w917) -> (x+1=w918:u64)
                          n466 = local write "Num_hits"(w918) -> ()
                        }
                        frame True {
                          n467 = local read "Num_hits"() -> (w920:u64)
                          n468 = Increment(x=w920) -> (x+1=w919:u64)
                          n469 = local write "Num_hits"(w919) -> ()
                        }
                      }
                      n470 = Subtract(x=w909, y="Вычет для \"антиразгона\"") -> (x-y=w910:dbl)
                      n471 = Equal?(x=w913, y=1) -> (x = y?=w907:bool)
                      n472 = And(x=w899, y=w907) -> (x .and. y?=w906:bool)
                      n473 = local write "ThRes value"(w915) -> ()
                      n474 = Select(t=w910, s=w906, f=w909) -> (s? t:f=w908:dbl)
                      n475 = local read "Num_hits_req"() -> (w904:u64)
                      n476 = local read "Num_hits"() -> (w905:u64)
                      n477 = Greater Or Equal?(x=w905, y=w904) -> (x >= y?=w903:bool)
                      n478 = Select(t=TRUE, s=w903, f=FALSE) -> (s? t:f=→"Стабилизировано":bool)
                    }
                  }
                }
              }
            }
          }
          n479 = Greater Or Equal?(x=w847, y=50) -> (x >= y?=w849:bool)
          n480 = case shown="False" w849 {
            tunnel: ["" "Too much try"] -> w837
            tunnel: [w922 TRUE] -> w848
            tunnel: w838 -> [w922 _]
            frame False {
            }
            frame True {
            }
          }
        }
        "Error message" <- w827
        n481 = local write "Подстроенное напряжение\nстабилизации"(w815) -> ()
        "NoStab" <- FALSE ("NoStab")
      }
    }
  }
  n482 = while {
    tunnel: w6 -> [w926]
    stop <- FALSE stop-if-true
    n483 = event shown="[0] \"stop\": Value Change" {
      selector: _ -> [_ _ _ _]
      dyn-events: _ -> [_ _ _ _]
      timeout: _ -> [_ _ _ _]
      tunnel: w926 -> [_ _ _ _]
      event "stop": Value Change {
        # "Работает, зараза, через раз"
        n484 = event-data() -> ()  [unwired: 1 in, 6 out]
        n485 = flat-sequence {
          frame #0 {
            n486 = local write "Case"(T1."Quit" ("Case")) -> ()
          }
          frame #1 {
            n487 = local write "stop"(FALSE) -> ()
            "Прервать" <- TRUE
          }
        }
      }
      event "Раб. режим LD": Value Change {
        n488 = event-data() -> ()  [unwired: 1 in, 6 out]
        n489 = flat-sequence {
          frame #0 {
            n490 = local write "Раб. режим LD"(FALSE) -> ()
            n491 = local write "Case"(T1."Bias" ("Case")) -> ()
          }
          frame #1 {
            n492 = local write "Выполняется"(TRUE) -> ()
          }
        }
      }
      event "Хар-ка TEC": Value Change {
        n493 = event-data() -> ()  [unwired: 1 in, 6 out]
        n494 = flat-sequence {
          frame #0 {
            n495 = local write "Хар-ка TEC"(FALSE) -> ()
            n496 = local write "Case"(T1."TEC_Chars" ("Case")) -> ()
          }
          frame #1 {
            n497 = local write "Выполняется"(TRUE) -> ()
          }
        }
      }
      event "Хар-ки от I_LD": Value Change {
        n498 = event-data() -> ()  [unwired: 1 in, 6 out]
        n499 = flat-sequence {
          frame #0 {
            n500 = local write "Хар-ки от I_LD"(FALSE) -> ()
            n501 = local write "Case"(T1."Characteristics" ("Case")) -> ()
          }
          frame #1 {
            n502 = local write "Выполняется"(TRUE) -> ()
          }
        }
      }
    }
  }
  n503 = while {
    tunnel: w5 -> [w940]
    tunnel: w3 -> [w941]
    stop <- FALSE stop-if-true
    w943 = T1."Initialization"  # Case
    n504 = disable-structure shown="Enabled" {
      frame Disabled {
        n505 = local read "Выполняется"() -> (w945:bool)
        n506 = Compound Arithmetic op=OR(w945) -> ()  [unwired: 1 in, 1 out]
      }
      frame Enabled {
      }
    }
    n507 = local read "Case"() -> (w942:T1)
    n508 = Equal?(x=w942, y=w943) -> (x = y?=w939:bool)
    n509 = case shown="False" w939 {
      tunnel: w941 -> [w947 _]
      tunnel: w940 -> [w946 _]
      frame False {
        n510 = stacked-sequence {
          tunnel: w947 -> [w952 w985 _ _ _]
          tunnel: w946 -> [w951 w984 _ w994 _]
          frame #0 {
            n511 = local read "Power Enable"() -> (w948:bool)
            n512 = call <instrlib>:"niDCPower Configure Output Enabled.vi"("output enabled"=w948, "channel name"="0,1,2", "instrument handle"=w952) -> ()  [unwired: 7 in, 2 out]
            n513 = call <instrlib>:"niDCPower Configure Output Enabled.vi"("output enabled"=w948, "channel name"="0,1,2", "instrument handle"=w951) -> ()  [unwired: 7 in, 2 out]
          }
          frame #1 {
            w964 = "1"
            w968 = 1000.0 ("y")
            w975 = "0" ("channel name")
            n514 = Divide(x="Предел тока ТЕС, мА", y=1000.0) -> (x/y=w978:dbl)
            n515 = call <instrlib>:"niDCPower Configure Current Limit.vi"("current limit"=w978, "channel name"="2", "instrument handle"=w985) -> ("instrument handle out"=w957:refnum<k15>)  [unwired: 7 in, 1 out]
            n516 = call <instrlib>:"niDCPower Configure Current Limit.vi"("current limit"=w978, "channel name"="0", "instrument handle"=w984) -> ("instrument handle out"=w971:refnum<k15>)  [unwired: 7 in, 1 out]
            n517 = Divide(x="Предел тока LD, мА", y=w968) -> (x/y=w979:dbl)
            n518 = Divide(x="Предел тока PDext, мА", y=w968) -> (x/y=w970:dbl)
            n519 = call <instrlib>:"niDCPower Configure Current Limit.vi"("current limit"=w970, "channel name"=w964, "instrument handle"=w971) -> ("instrument handle out"=w963:refnum<k15>)  [unwired: 7 in, 1 out]
            n520 = call <instrlib>:"niDCPower Measure Multiple.vi"("channel name"="2", "instrument handle"=w957) -> ("current measurements"=w960:dbl[])  [unwired: 6 in, 3 out]
            n521 = call <instrlib>:"niDCPower Configure Current Limit.vi"("current limit"=w979, "channel name"=w975, "instrument handle"=w957) -> ("instrument handle out"=w976:refnum<k15>)  [unwired: 7 in, 1 out]
            n522 = call <instrlib>:"niDCPower Measure Multiple.vi"("channel name"=w964, "instrument handle"=w963) -> ("current measurements"=w965:dbl[])  [unwired: 6 in, 3 out]
            n523 = Index Array(array=w960) -> (element=w959:dbl)  [unwired: 1 in]
            n524 = call <instrlib>:"niDCPower Measure Multiple.vi"("channel name"=w975, "instrument handle"=w976) -> ("current measurements"=w974:dbl[])  [unwired: 6 in, 3 out]
            n525 = Multiply(x=w959, y=1000.0) -> (x*y=w961:dbl)
            n526 = Index Array(array=w965) -> (element=w966:dbl)  [unwired: 1 in]
            n527 = Absolute Value(x=w961) -> (abs(x)=w955:dbl)
            n528 = Index Array(array=w974) -> (element=w973:dbl)  [unwired: 1 in]
            n529 = Multiply(x=w966, y=1000.0) -> (x*y=w962:dbl)
            n530 = local write "TEC_current, mA"(w955) -> ()
            n531 = Absolute Value(x=w962) -> (abs(x)=w953:dbl)
            "IPD, mA" <- w953
            n532 = Multiply(x=w973, y=1000.0) -> (x*y=w954:dbl)
            "Operating Current" <- w954
            n533 = local write "Operating Current, mA"(w954) -> ()
            n534 = local write "IPD(ext), mA"(w953) -> ()
          }
          frame #2 {
            n535 = Wait (ms)(milliseconds to wait=u32 100) -> ()  [unwired: 1 out]
            n536 = case shown="True" "Принудительная стабилизация" {
              frame False {
              }
              frame True {
                n537 = stacked-sequence {
                  frame #0 {
                    n538 = local read "Num_hits_req"() -> (w988:u64)
                    n539 = local write "Num_hits"(w988) -> ()
                  }
                  frame #1 {
                    n540 = local write "Принудительная стабилизация"(FALSE) -> ()
                  }
                }
              }
            }
          }
          frame #3 {
            # "Полярность пельтье"
            n541 = Select(t=0.0, s="Нагрев", f=-5.0) -> (s? t:f=w990:dbl)
            n542 = call <instrlib>:"niDCPower Configure Voltage Level.vi"("voltage level"=w990, "channel name"="2", "instrument handle"=w994) -> ()  [unwired: 7 in, 2 out]
          }
          frame #4 {
            w1002 = T4 7.5 items=["3 1/2"=3.5, "4 1/2"=4.5, "5 1/2"=5.5, "6 1/2"=6.5, "7 1/2"=7.5] ("Resolution in Digits")
            n543 = local read "4071(1)_adress"() -> (w1003:refnum<k15>)
            n544 = call-poly <instrlib>:"niDMM Config Measurement.vi"("Range"=-1.0 ("Configuration:Measurement Options:Max Frequency"), "Resolution in Digits"=w1002, "Function"=niDMM_Function."DC Current" ("multimeter mode"), "instrument handle"=w1003) -> ("instrument handle out"=w1001:refnum<k15>)  [unwired: 6 in, 1 out]
            n545 = for {
              N: 5 -> [_]
              tunnel: w1001 -> [w1009]
              tunnel: [w1006] -> w997 mode=indexing
              n546 = call <instrlib>:"niDMM Read.vi"("instrument handle"=w1009) -> ("Measurement"=w1007:dbl)  [unwired: 8 in, 2 out]
              n547 = Absolute Value(x=w1007) -> (abs(x)=w1006:dbl)
              n548 = Wait (ms)(milliseconds to wait=u32 50) -> ()  [unwired: 1 out]
            }
            n549 = call-poly <vilib>:"Mean.vi"("X"=w997) -> ("mean"=w998:dbl)  [unwired: 1 out]
            n550 = Multiply(x=w998, y=1000000.0) -> (x*y=→"Monitor Current, uA":dbl)
          }
        }
      }
      frame True {
        n551 = Wait (ms)(milliseconds to wait=u32 20) -> ()  [unwired: 1 out]
      }
    }
  }
  n552 = while {
    tunnel: w3 -> [w1012]
    tunnel: w5 -> [w1011]
    stop <- FALSE stop-if-true
    n553 = local read "stop"() -> (w1013:bool)
    n554 = case shown="False" w1013 {
      tunnel: w1012 -> [_ w1016]
      tunnel: w1011 -> [_ w1015]
      frame False {
      }
      frame True {
        n555 = stacked-sequence {
          tunnel: w1016 -> [_ _ _ _ w1035 _]
          tunnel: w1015 -> [_ _ _ _ w1034 _]
          frame #0 {
            w1017 = T1."Initialization"  # Case
            n556 = local write "Case"(w1017) -> ()
          }
          frame #1 {
            # "Закрытие логов"
            n557 = property on="Op(Ild)_Log_address" class="Ref (strict)"() -> ("Value"=w1021:refnum<file>)  [unwired: 2 in, 2 out]
            n558 = property on="Param_Log_address" class="Ref (strict)"() -> ("Value"=w1022:refnum<file>)  [unwired: 2 in, 2 out]
            n559 = property on="V2(Ild)_Log_address" class="Ref (strict)"() -> ("Value"=w1020:refnum<file>)  [unwired: 2 in, 2 out]
            n560 = Format Into String(initial string=w1021, "\r\n") -> (resulting string=w1031:refnum<file>)  [unwired: 2 in, 1 out]
            n561 = Format Into String(initial string=w1022, "\r\n") -> (resulting string=w1030:refnum<file>)  [unwired: 2 in, 1 out]
            n562 = Format Into String(initial string=w1020, "\r\n") -> (resulting string=w1028:refnum<file>)  [unwired: 2 in, 1 out]
            n563 = Close File(refnum=w1031) -> ()  [unwired: 1 in, 2 out]
            n564 = Close File(refnum=w1030) -> ()  [unwired: 1 in, 2 out]
            n565 = Close File(refnum=w1028) -> ()  [unwired: 1 in, 2 out]
            n566 = property on="Ipd(Ild)_Monitor_Log_address" class="Ref (strict)"() -> ("Value"=w1018:refnum<file>)  [unwired: 2 in, 2 out]
            n567 = property on="Ipd(Ild)_External_Log_address" class="Ref (strict)"() -> ("Value"=w1019:refnum<file>)  [unwired: 2 in, 2 out]
            n568 = Format Into String(initial string=w1019, "\r\n") -> (resulting string=w1025:refnum<file>)  [unwired: 2 in, 1 out]
            n569 = Format Into String(initial string=w1018, "\r\n") -> (resulting string=w1024:refnum<file>)  [unwired: 2 in, 1 out]
            n570 = Close File(refnum=w1025) -> ()  [unwired: 1 in, 2 out]
            n571 = Close File(refnum=w1024) -> ()  [unwired: 1 in, 2 out]
          }
          frame #2 {
            # "Выключение Офира"
          }
          frame #3 {
            w1033 = FALSE
            n572 = local write "Раб. режим LD"(w1033) -> ()
            n573 = local write "Хар-ки от I_LD"(w1033) -> ()
            n574 = local write "Power Enable"(w1033) -> ()
            n575 = local write "Хар-ка TEC"(w1033) -> ()
          }
          frame #4 {
            w1038 = "0,1,2" ("channel name")
            w1043 = "0,1,2" ("channel name")
            n576 = call <instrlib>:"niDCPower Configure Voltage Level.vi"("voltage level"=0.0, "channel name"=w1043, "instrument handle"=w1035) -> ("instrument handle out"=w1042:refnum<k15>)  [unwired: 7 in, 1 out]
            n577 = call <instrlib>:"niDCPower Configure Voltage Level.vi"("voltage level"=0.0, "channel name"=w1038, "instrument handle"=w1034) -> ("instrument handle out"=w1039:refnum<k15>)  [unwired: 7 in, 1 out]
            n578 = call <instrlib>:"niDCPower Configure Output Enabled.vi"("output enabled"=FALSE, "channel name"=w1043, "instrument handle"=w1042) -> ("instrument handle out"=w1041:refnum<k15>)  [unwired: 7 in, 1 out]
            n579 = call <instrlib>:"niDCPower Configure Output Enabled.vi"("output enabled"=FALSE, "channel name"=w1038, "instrument handle"=w1039) -> ("instrument handle out"=w1040:refnum<k15>)  [unwired: 7 in, 1 out]
            n580 = call <instrlib>:"niDCPower Close.vi"("instrument handle"=w1041) -> ()  [unwired: 10 in, 1 out]
            n581 = call <instrlib>:"niDCPower Close.vi"("instrument handle"=w1040) -> ()  [unwired: 10 in, 1 out]
          }
          frame #5 {
            n582 = Stop(stop? (T)=TRUE) -> ()
          }
        }
      }
    }
  }
  n583 = disable-structure shown="Disabled" {
    frame Disabled {
      n584 = local read "4070_address"() -> (w1050:refnum<k15>)
      n585 = local read "TEC_Source"() -> (w1047:enum16{"S1_Ch2", "S2_Ch0", "S3_Ch1"})
      n586 = case shown="\"S3_Ch1\"" w1047 {
        tunnel: [w1060 w1062 w1064] -> w1049
        tunnel: ["2" "0" "1"] -> w1048
        frame "S1_Ch2", Default {
          n587 = local read "Source_1_Vcc_out"() -> (w1060:refnum<k15>)
        }
        frame "S2_Ch0" {
          n588 = local read "Source_2_Vcc_out"() -> (w1062:refnum<k15>)
        }
        frame "S3_Ch1" {
          n589 = local read "Source_3_Vcc_out"() -> (w1064:refnum<k15>)
        }
      }
      n590 = call "Res_stabiliz.vi"("Точность ThRes"="Точность ThRes", "Up_Volt_limit"="the upper limit for the voltage", "Optimum ThRes"="Optimum ThRes", "Low_Volt_limit"="the lower limit for the voltage", "TEC_Source"=w1049, "4070_address"=w1050, "channel name"=w1048) -> ("Подстроенное напряжение"=→"Подстроенное напряжение\nстабилизации":dbl, "ThRes value"=→"ThRes value":dbl, "thRes_adj"=w1058:dbl, "Start Voltage"=w1051:dbl)  [unwired: 1 out]
      n591 = local write "Сопротивление терморез-ра"(w1058) -> ()
    }
    frame Enabled {
    }
  }
  n592 = disable-structure shown="Enabled" {
    frame Disabled {
      # "Есть в инициализации"
      # "Для измерения Сопротивления"
      # "Поменять in0/in1 для ТЕС"
      n593 = local read "Source_2_Vcc_out"() -> (w1070:refnum<k15>)
      n594 = local read "4070_Rele_source"() -> (w1065:enum16{"S2_Ch0", "S1_Ch2"})
      n595 = call <instrlib>:"niDCPower Configure Voltage Level.vi"("voltage level"=-5.0, "channel name"="2", "instrument handle"=w1070) -> ()  [unwired: 7 in, 2 out]
      n596 = case shown="\"S1_Ch2\"" w1065 {
        tunnel: [5.0 -5.0] -> w1066
        tunnel: ["0" "2"] -> w1067
        tunnel: [w1072 w1075] -> w1068
        frame "S2_Ch0", Default {
          n597 = local read "Source_2_Vcc_out"() -> (w1072:refnum<k15>)
        }
        frame "S1_Ch2" {
          n598 = local read "Source_1_Vcc_out"() -> (w1075:refnum<k15>)
        }
      }
      n599 = call <instrlib>:"niDCPower Configure Voltage Level.vi"("voltage level"=w1066, "channel name"=w1067, "instrument handle"=w1068) -> ()  [unwired: 7 in, 2 out]
    }
    frame Enabled {
    }
  }
  "Выполняется" <- w4
